vi "Trajectory Builder.vi"() -> ()   [LabVIEW 2019]
uses:
  Command Stuff/Command Editor Info.ctl
  Command Stuff/Single Cmd Info.ctl
  <vilib>/picture/picture.llb/imagedata.ctl
  <vilib>/Utility/miscctls.llb/LVPositionTypeDef.ctl
  Command Stuff/Availible Command systems for auto.ctl
  <vilib>/event_ctls.llb/lveventtype.ctl
panel:
  in  "Cluster":T1={"Path Backwards"=TRUE, "Robot Backwards"=TRUE}
  in  "Zero Vel":bool
  out "Picture":picture
  out "Duration (s)":dbl format="%#.4g"
  out "Distance (ft)":dbl format="%#.1g"
  in  "Instructions":string="Directions:\nUse mouse to ...\n    move robot position (rectangle with arrow)\n    rotate robot (red arrow)\n    move waypoints (numbered circles)\nClick in open space to add a waypoint\nShift click to delete a waypoint\nHover over a waypoint and use arrow keys to nudge\n\nTime slider and Play button will run robot along path to test for collisions.\n\nDirection and Destionation are folder selectors for files\n\nNew creates a new path at default location\n\nAppend creates a path using current path's position and heading.\n\nTo add a command, move robot using Time slider and double click Command in Palette.\n\nYou can modify command timing in the graph or Command Sequencer tree.\n\nEnable/disable a command by clicking on the enable column item.\n\nDelete a command by shift-clicking in the enable column.\n\nTo configure command parameters, Select the command name in the tree, Open Panel, enter parameters, and Inhale the parameters."
  out "WayPoints":cluster{"x":dbl, "y":dbl, "th":dbl}[](array[cluster]) {"th" format="%#_4g"}
  in  "Scale Factor":dbl=0.75
  out "Command Palette":picture
  in  "Cache":T5
  out "folder names":cluster{"name":string, "name":string}
  in  "Directory":bool
  in  "Tab Control":T6(tab)
  in  "Center Flip":bool
  in  "Snap to foot":bool
  in  "Angle Limiter":enum16{"90", "45", "15", "1"}(ring)=enum."15"
  in  "Snap robot to baseline":bool
  in  "Acceleration Overrides":T7 {"Angular \nAccelerations" step=5.0}
  in  "Sample Period (s)":dbl=0.02 format="%#_6p"
  in  "Limits":T8={"Velocity (fps)"=6.0, "Accel (fps^2)"=15.0, "Jerk (fps^3)"=150.0} {"Jerk (fps^3)" min=0.0 step=1.0; "Accel (fps^2)" min=0.0; "Velocity (fps)" min=0.0}
  in  "Conditions":T9 {"vFinal (fps)" min=0.0; "vInitial (fps)" min=0.0}
  in  "Unjank":bool
  in  "Turn Acceleration":bool=TRUE
  in  "Turn Deceleration":bool=TRUE
  in  "Open Command":bool
  in  "Inhale":bool
  in  "Command Sequence":string(tree)
  in  "Projects":u16(ring)
  in  "Refresh":bool
  in  "Time (s)":dbl(slide) scale=0.0..3.16 scale format="%#.1g"
  in  "Play":bool
  in  "Sub Dir 2":u16(ring)
  in  "Sub Dir 1":u16(ring) items=["Experimental", "Real Paths"]
  out "fps":dbl[](graph)
  in  "Append":bool
  in  "Open":i32(listbox)
  in  "Filename":string
  in  "Save":bool
  in  "New":bool
  # "Command Palette"
  # "Power Port"
  # "Feeder Station"
  # "Nicotine"
  # "Interaction Options"
  # "1"
  # "2"
  # "3"
  # "4"
  # "5"
  # "6"
  # "7"
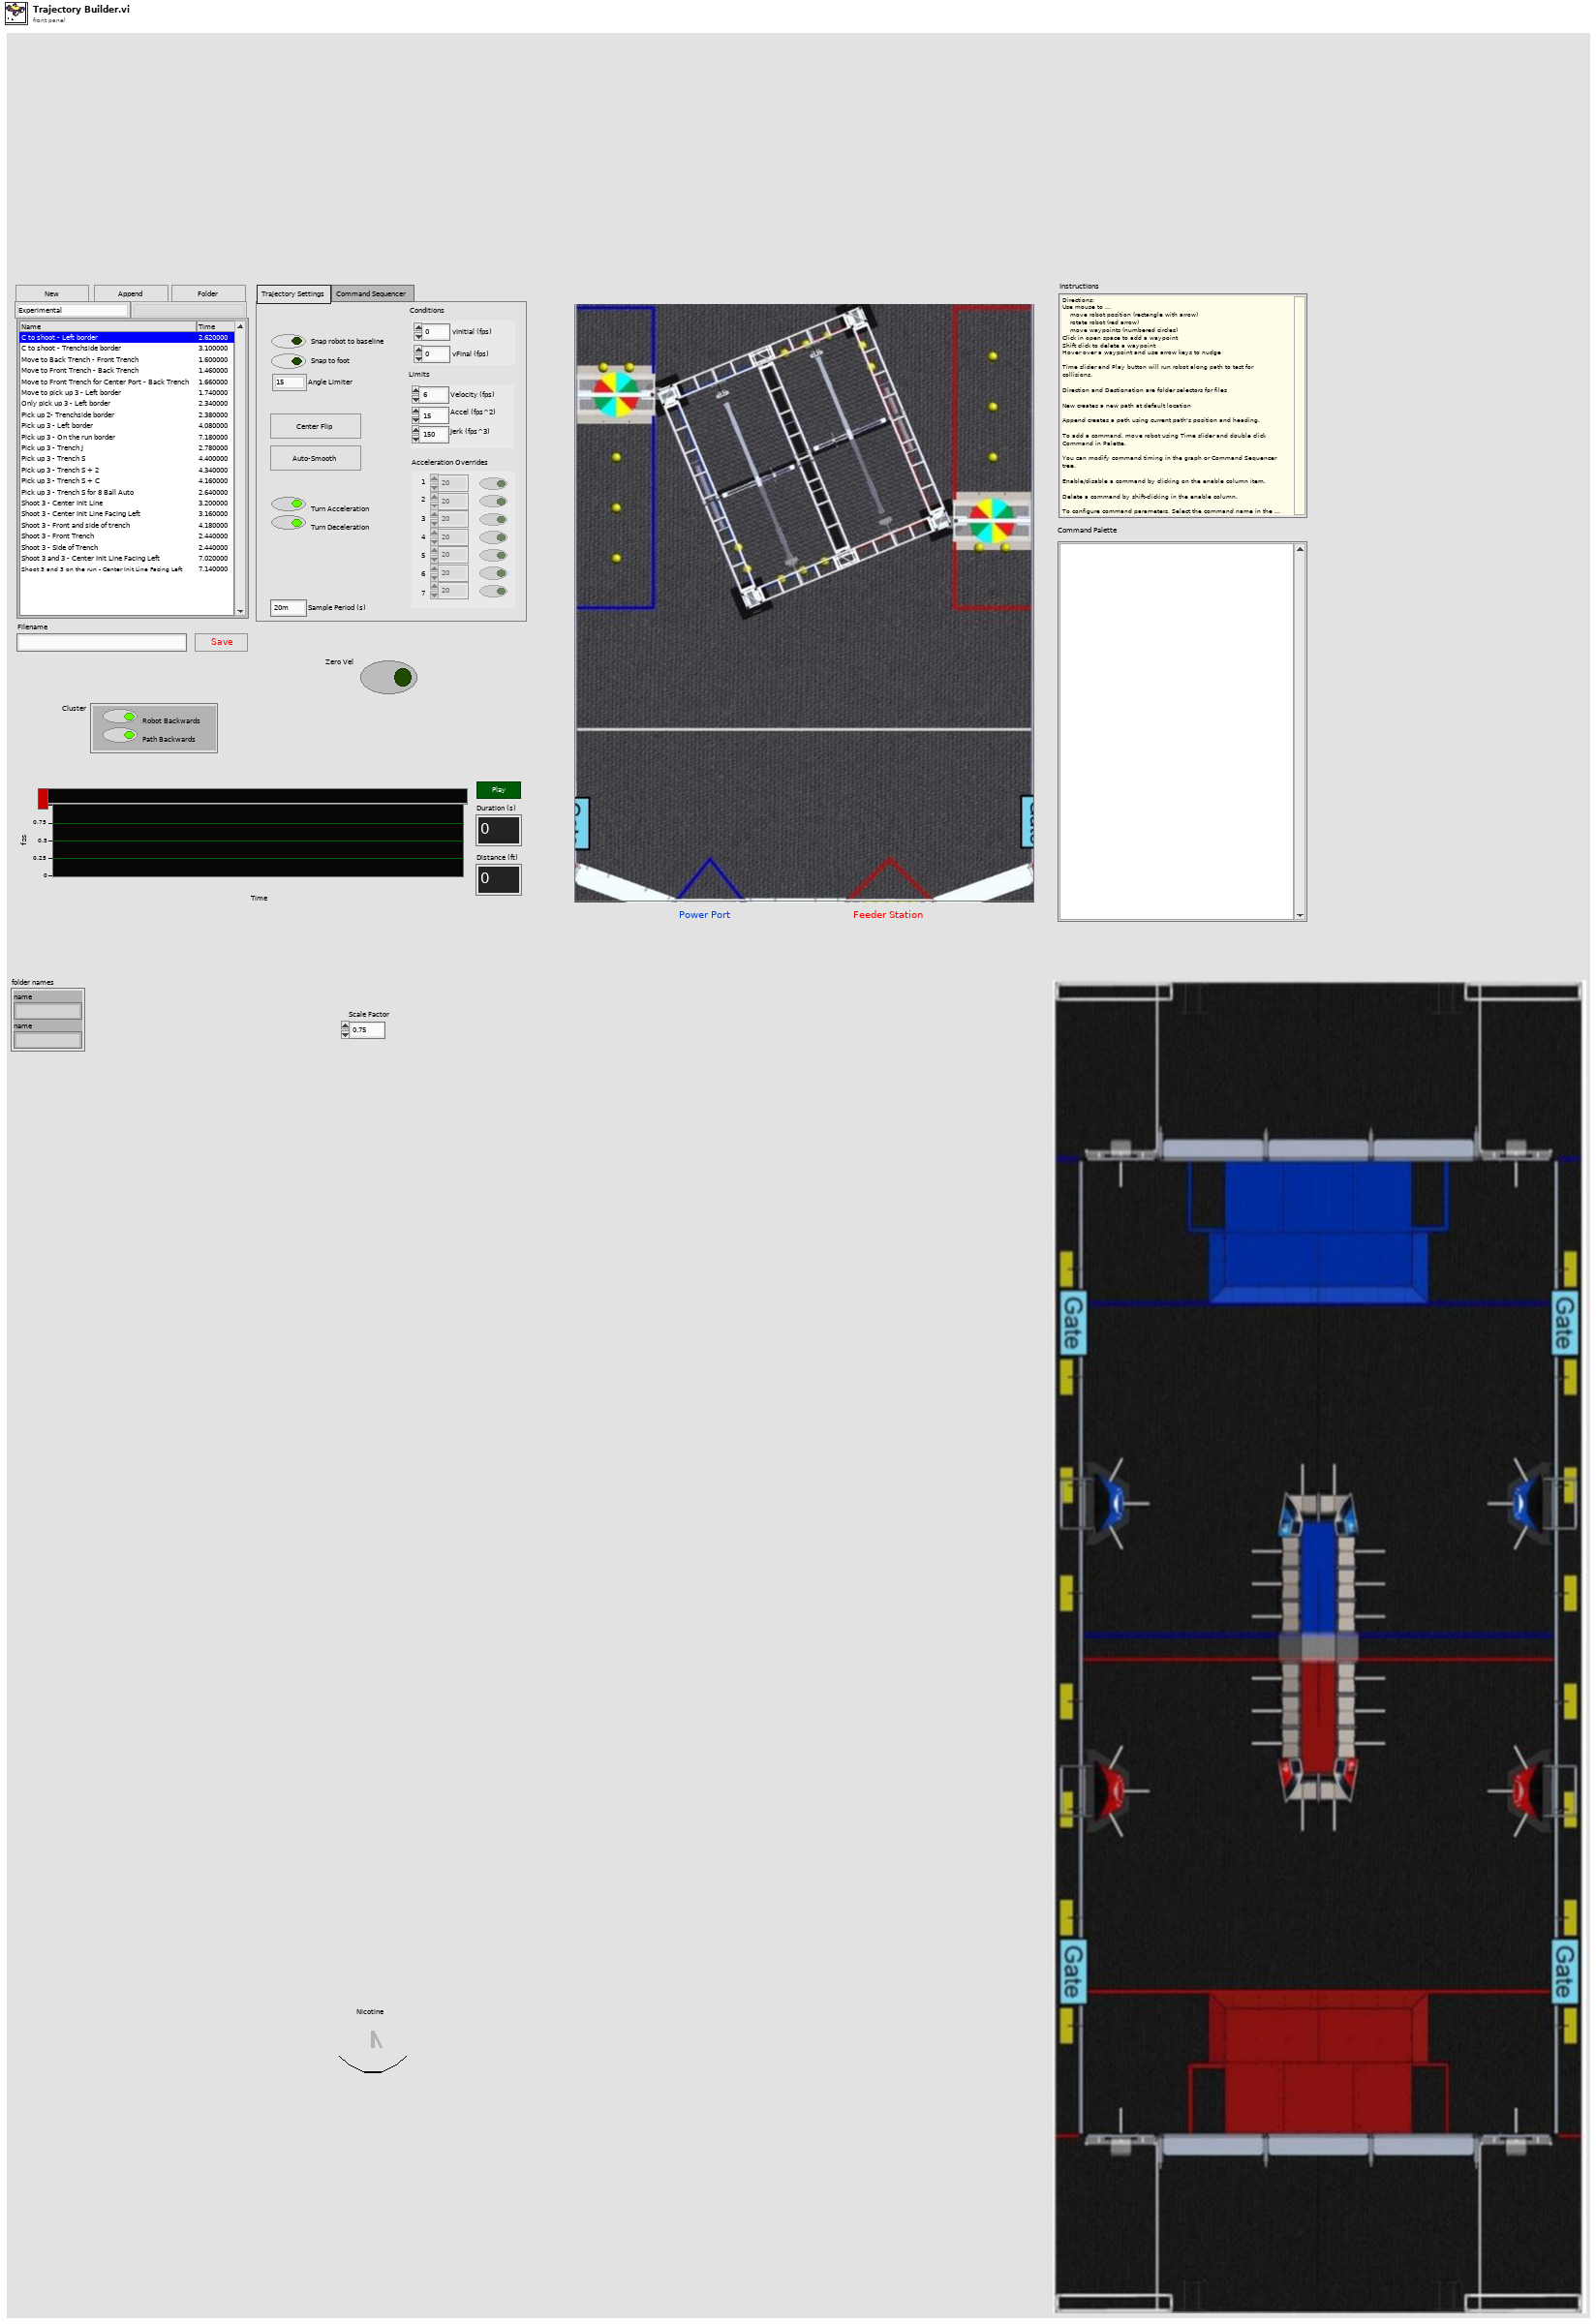
[diagram p1: front panel]
types:
  T1 = cluster{"Path Backwards":bool, "Robot Backwards":bool}
  T2 = typedef "Command Editor Info.ctl" = T3[]
  T3 = typedef "Single Cmd Info.ctl" = cluster{"Name":string, "CPTM.DataType":variant, "All Control Values Variant":cluster{"Name":string, "Variant Data":variant}[], "icon full":T4, "icon scaled":T4, "Path":path, "Subsystem Color":u32}
  T4 = typedef "imagedata.ctl" = cluster{"image type":i32, "image depth":i32, "image":u8[], "mask":u8[], "colors":u32[], "Rectangle":cluster{"left":i16, "top":i16, "right":i16, "bottom":i16}}
  T5 = cluster{"Filtered Command Info Out":T2, "2D Picture":picture}
  T6 = enum32{"Trajectory Settings", "Command Sequencer"}
  T7 = cluster{"Angular \nAccelerations":dbl[], "Accel Override Bools":bool[]}
  T8 = cluster{"Velocity (fps)":dbl, "Accel (fps^2)":dbl, "Jerk (fps^3)":dbl}
  T9 = cluster{"vInitial (fps)":dbl, "vFinal (fps)":dbl}
  T10 = typedef "LVPositionTypeDef.ctl" = cluster{"Left":i32, "Top":i32}
  T11 = cluster{"Sample Period (s)":dbl, "Limits":cluster{"Velocity (fps)":dbl, "Acceleration (fps^2)":dbl, "Jerk (fps^3)":dbl}, "Conditions":cluster{"vInitial (fps)":dbl, "vFinal (fps)":dbl}, "output cluster":cluster{"Angular \nAccelerations":dbl[], "Override Limits?":bool[]}}
  T12 = cluster{"Segment Name":string, "Type":enum16{"Accel Straight", "Const Straight", "Blend", "Circle"}, "Traj Pos Points":cluster{"x":dbl, "y":dbl, "th":dbl}[], "Traj Vel Points":cluster{"V":dbl, "th":dbl}[], "Accel Index":i32, "Decel Index":i32}[]
  T13 = cluster{"Angular \nAccelerations":dbl[], "Override Limits?":bool[]}
  T14 = cluster{"Index":i32, "Pt Test Results":enum16{"Miss", "Rect Hit", "Arrow Hit"}}
  T15 = cluster{"Drag Object":cluster{"Index":i32, "x":dbl, "y":dbl}, "Hover Object":cluster{"Index":i32, "Pt Test Results":enum16{"Miss", "Rect Hit", "Arrow Hit"}}, "Filename":string}
  T16 = cluster{"Trajectory Data":cluster{"Segment Name":string, "Type":enum16{"Accel Straight", "Const Straight", "Blend", "Circle"}, "Traj Pos Points":cluster{"x":dbl, "y":dbl, "th":dbl}[], "Traj Vel Points":cluster{"V":dbl, "th":dbl}[], "Accel Index":i32, "Decel Index":i32}[], "Points":cluster{"x":dbl, "y":dbl, "th":dbl}[], "Cluster":cluster{"Sample Period (s)":dbl, "Limits":cluster{"Velocity (fps)":dbl, "Acceleration (fps^2)":dbl, "Jerk (fps^3)":dbl}, "Conditions":cluster{"vInitial (fps)":dbl, "vFinal (fps)":dbl}, "output cluster":cluster{"Angular \nAccelerations":dbl[], "Override Limits?":bool[]}}, cluster{"Time (s)":dbl, T3, bool}[]}
  T17 = cluster{"Velocity":dbl, "Sample Time":dbl, "Accel":dbl}
  T18 = cluster{"Sample Period (s)":dbl, "Limits":cluster{"Velocity (fps)":dbl, "Acceleration (fps^2)":dbl, "Jerk (fps^3)":dbl}, "Conditions":cluster{"vInitial (fps)":dbl, "vFinal (fps)":dbl}}
  T19 = cluster{"Sample Period (s)":dbl, "Limits":cluster{"Velocity (fps)":dbl, "Acceleration (fps^2)":dbl, "Jerk (fps^3)":dbl}, "Conditions":cluster{"vInitial (fps)":dbl, "vFinal (fps)":dbl}, "Min Rads":dbl[]}
  T20 = typedef "Availible Command systems for auto.ctl" = u16
  T21 = cluster{"Time into Path":dbl, "System":T20, "Item Selected?":bool, "System Selection":T20}[]
  T22 = typedef "lveventtype.ctl" = enum32{"Null", "Timeout", "Annotation Menu Selection", "Annotation Menu Selection?", "App Instance Close", "App Instance Close?", "Autoscale Range Change", "Bookmark Info Change", "Cell Edit", "Cell Edit?", "Cursor Grab", "Cursor Grab?", "Cursor Menu Selection", "Cursor Menu Selection?", "Cursor Move", "Cursor Release", "Data Change", "Direction Change", "Display State Change", "Drag Ended", "Drag Enter", "Drag Leave", "Drag Over", "Drag Source Update", "Drag Starting", "Drag Starting?", "Drop", "Exec State Change", "Key Down", "Key Down?", "Key Repeat", "Key Repeat?", "Key Up", "Listbox Double Click", "Menu Activation?", "Menu Selection (App)", "Menu Selection? (App)", "Menu Selection (User)", "Mouse Down", "Mouse Down?", "Mouse Enter", "Mouse Leave", "Mouse Move", "Mouse Up", "Mouse Wheel", "NI Security User Change (App)", "Pane Size", "Panel Close", "Panel Close?", "Panel Resize", "Plot Attribute Change", "Scale Range Change", "Shortcut Menu Activation?", "Shortcut Menu Selection (App)", "Shortcut Menu Selection? (App)", "Shortcut Menu Selection (User)", "Tree Double Click", "Tree Drag", "Tree Drag?", "Tree Drop", "Tree Drop?", "Tree Item Close", "Tree Item Close?", "Tree Item Open", "Tree Item Open?", "User Event", "Value Change"}
  T23 = enum32{"Invalid", "Standard", "Closed", "Hidden", "Minimized", "Maximized"}
  T24 = cluster{"Sample Period (s)":dbl, "Limits":cluster{"Velocity (fps)":dbl, "Accel (fps^2)":dbl, "Jerk (fps^3)":dbl}, "Conditions":cluster{"vInitial (fps)":dbl, "vFinal (fps)":dbl}, " Acceleration Overrides":cluster{"Angular \nAccelerations":dbl[], "Accel Override Bools":bool[]}}
  T25 = cluster{"Segment Name":string, "Type":enum16{"Accel Straight", "Const Straight", "Blend", "Circle"}, "Traj Pos Points":cluster{"x":dbl, "y":dbl, "th":dbl}[], "Traj Vel Points":cluster{"V":dbl, "th":dbl}[], "Accel Index":i32, "Decel Index":i32}
  T26 = cluster{"Trajectory Data":cluster{"Segment Name":string, "Type":enum16{"Accel Straight", "Const Straight", "Blend", "Circle"}, "Traj Pos Points":cluster{"x":dbl, "y":dbl, "th":dbl}[], "Traj Vel Points":cluster{"V":dbl, "th":dbl}[], "Accel Index":i32, "Decel Index":i32}[], "Updated Waypoints":cluster{"x":dbl, "y":dbl, "th":dbl}[], "Cluster":cluster{"Sample Period (s)":dbl, "Limits":cluster{"Velocity (fps)":dbl, "Accel (fps^2)":dbl, "Jerk (fps^3)":dbl}, "Conditions":cluster{"vInitial (fps)":dbl, "vFinal (fps)":dbl}, " Acceleration Overrides":cluster{"Angular \nAccelerations":dbl[], "Accel Override Bools":bool[]}}, cluster{"Time (s)":dbl, T3, bool}[]}
  T27 = cluster{"Velocity":dbl, "Accel":dbl, "Accel":dbl}
  T28 = cluster{"Velocity (fps)":dbl, "Acceleration (fps^2)":dbl, "Jerk (fps^3)":dbl}
  T29 = cluster{"Trajectory Data":cluster{"Segment Name":string, "Type":enum16{"Accel Straight", "Const Straight", "Blend", "Circle"}, "Traj Pos Points":cluster{"x":dbl, "y":dbl, "th":dbl}[], "Traj Vel Points":cluster{"V":dbl, "th":dbl}[], "Accel Index":i32, "Decel Index":i32}[], "Points":cluster{"x":dbl, "y":dbl, "th":dbl}[], cluster{"Sample Period (s)":dbl, "Limits":cluster{"Velocity (fps)":dbl, "Accel (fps^2)":dbl, "Jerk (fps^3)":dbl}, "Conditions":cluster{"vInitial (fps)":dbl, "vFinal (fps)":dbl}, " Acceleration Overrides":cluster{"Angular \nAccelerations":dbl[], "Accel Override Bools":bool[]}}, cluster{"Time (s)":dbl, T3, bool}[]}
  T30 = typedef "LVPoint32TypeDef.ctl" = cluster{"Horizontal":i32, "Vertical":i32}
  T31 = cluster{"Shift":bool, "Ctrl":bool, "Alt":bool, "Cmd":bool, "Opt":bool}
  T32 = typedef "LVBoundsTypeDef.ctl" = cluster{"Width":u32, "Height":u32}
  T33 = cluster{"Snap robot to baseline":bool, "Snap to foot":bool, "Angle Limiter":enum16{"90", "45", "15", "1"}}
  T34 = cluster{i32, "Pt Test Results":enum16{"Miss", "Rect Hit", "Arrow Hit"}}
  T35 = typedef "eventvkey.ctl" = enum16{"ASCII", "Enter", "Return", "Shift", "Ctrl", "Alt", "Cmd", "Opt", "Caps", "NumLock", "Clear", "Break", "Up", "Down", "Left", "Right", "Insert", "Delete", "Home", "End", "PageUp", "PageDown", "Escape", "Help", "Pause", "ScrollLock", "F1", "F2", "F3", "F4", "F5", "F6", "F7", "F8", "F9", "F10", "F11", "F12", "F13", "F14", "F15", "F16", "F17", "F18", "F19", "F20", "F21", "F22", "F23", "F24", "Play", "VolumeUp", "VolumeDown", "Mute", "Two Byte Char"}
  T36 = cluster{"Name":string, "CPTM.DataType":variant, "Get All Control Values Variant":cluster{"Name":string, "Variant Data":variant}[], "Color 256":T4, "Subsystem Color":u32}[]
  T37 = cluster{"Trajectory Data":cluster{"Segment Name":string, "Type":enum16{"Accel Straight", "Const Straight", "Blend", "Circle"}, "Traj Pos Points":cluster{"x":dbl, "y":dbl, "th":dbl}[], "Traj Vel Points":cluster{"V":dbl, "th":dbl}[], "Accel Index":i32, "Decel Index":i32}[], "Updated Waypoints":cluster{"x":dbl, "y":dbl, "th":dbl}[], cluster{"Sample Period (s)":dbl, "Limits":cluster{"Velocity (fps)":dbl, "Accel (fps^2)":dbl, "Jerk (fps^3)":dbl}, "Conditions":cluster{"vInitial (fps)":dbl, "vFinal (fps)":dbl}, " Acceleration Overrides":cluster{"Angular \nAccelerations":dbl[], "Accel Override Bools":bool[]}}, cluster{"Time (s)":dbl, T3, bool}[]}
  T38 = cluster{"Horizontal":dbl, "Vertical":dbl, "th":dbl}
  T39 = cluster{"Name":string, "Color":u32, "Style":i32, "Point Style":i32, "Name Visible":bool, "Allow Drag":bool, "Annotation Mode":i32, "Plot":i32, "Index":i32, "Position":cluster{"X":dbl, "Y":dbl}, "X Scale":i32, "Y Scale":u32, "Show Arrow":bool, "Lock Name":bool, "Plot Area":i32, "Label Offset":cluster{"X":dbl, "Y":dbl}}[]
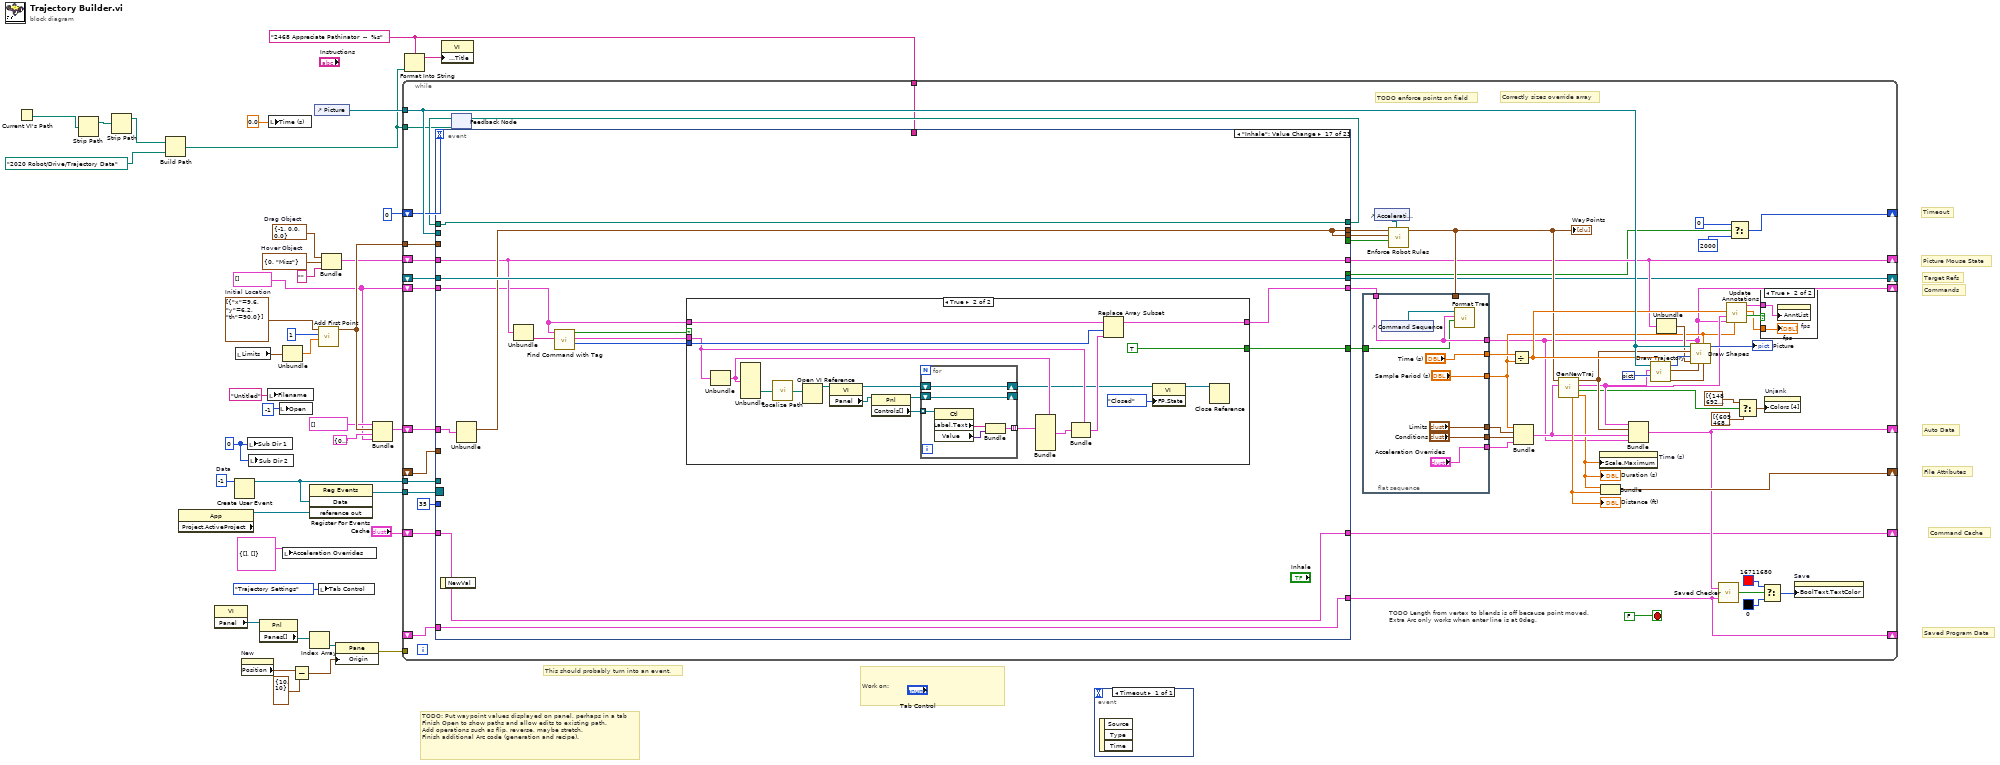
[diagram p0: block diagram]
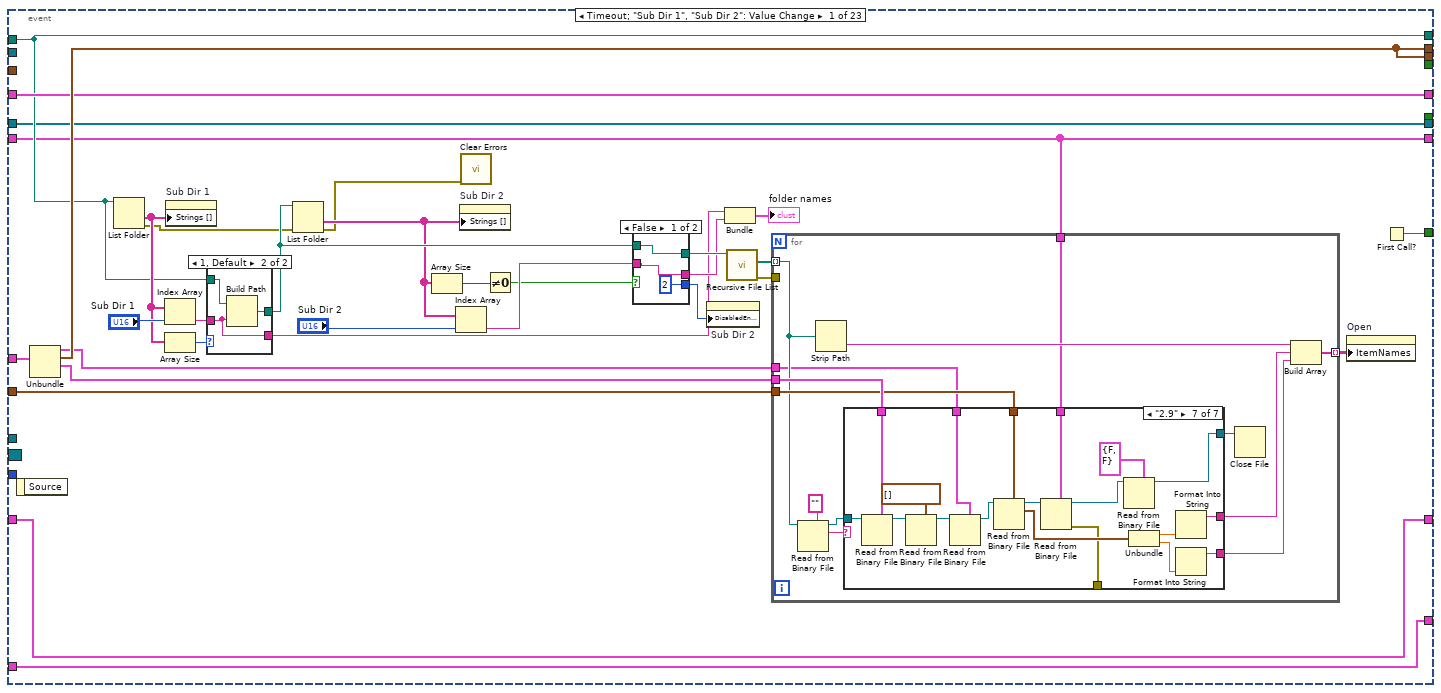
[diagram p3: hidden frame]
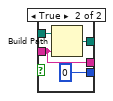
[diagram p5: hidden frame]
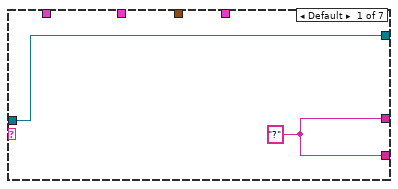
[diagram p6: hidden frame]
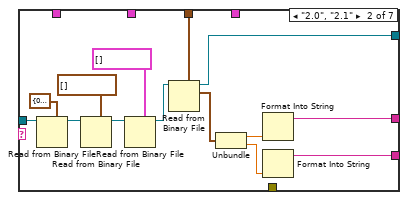
[diagram p7: hidden frame]
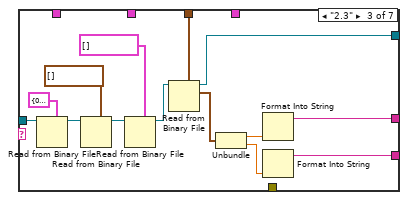
[diagram p8: hidden frame]
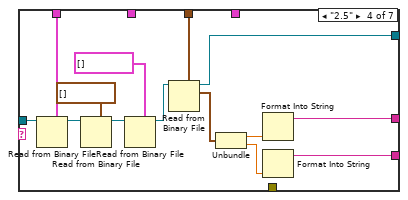
[diagram p9: hidden frame]
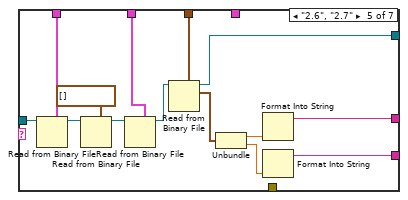
[diagram p10: hidden frame]
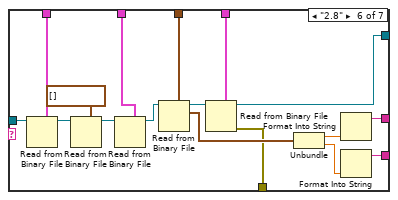
[diagram p11: hidden frame]
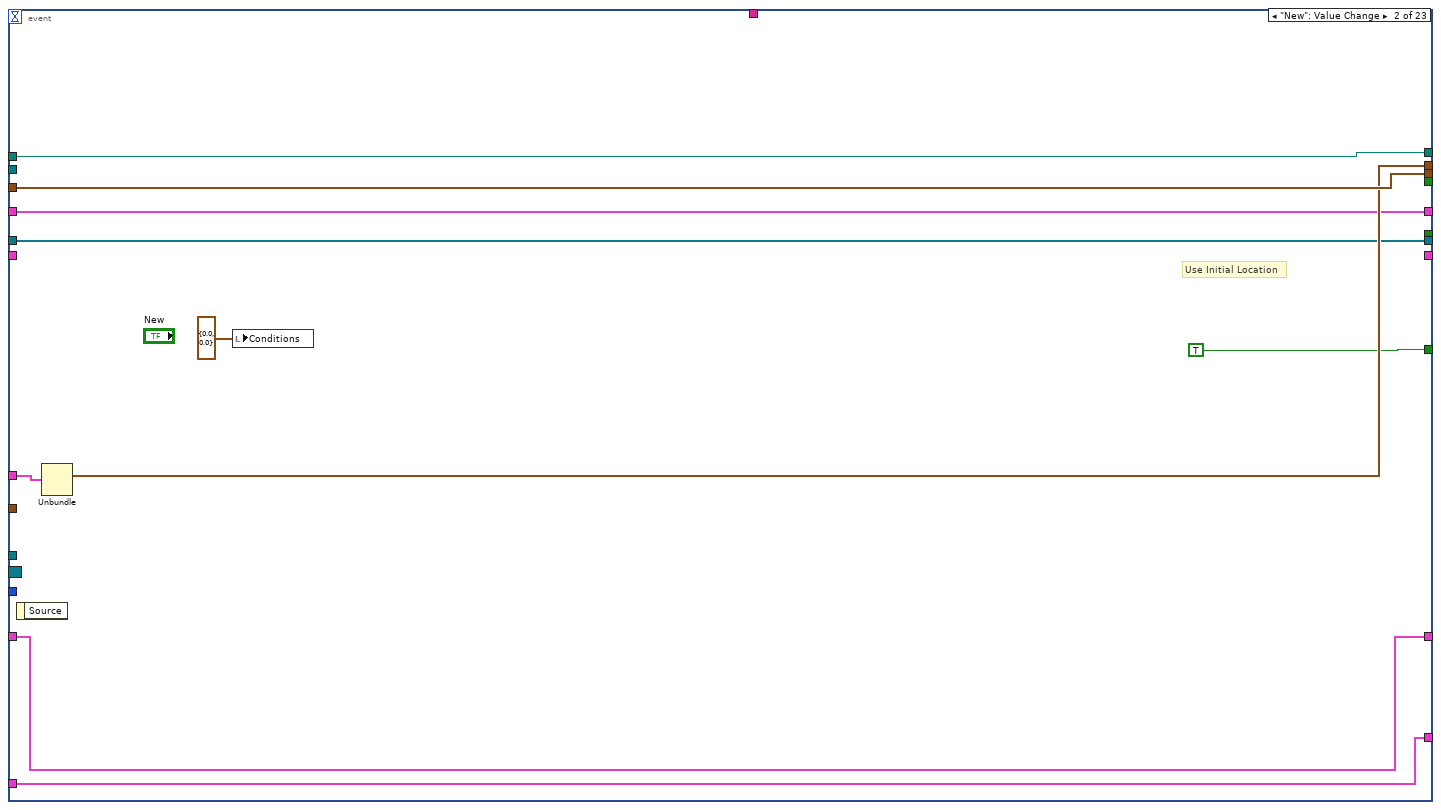
[diagram p12: hidden frame]
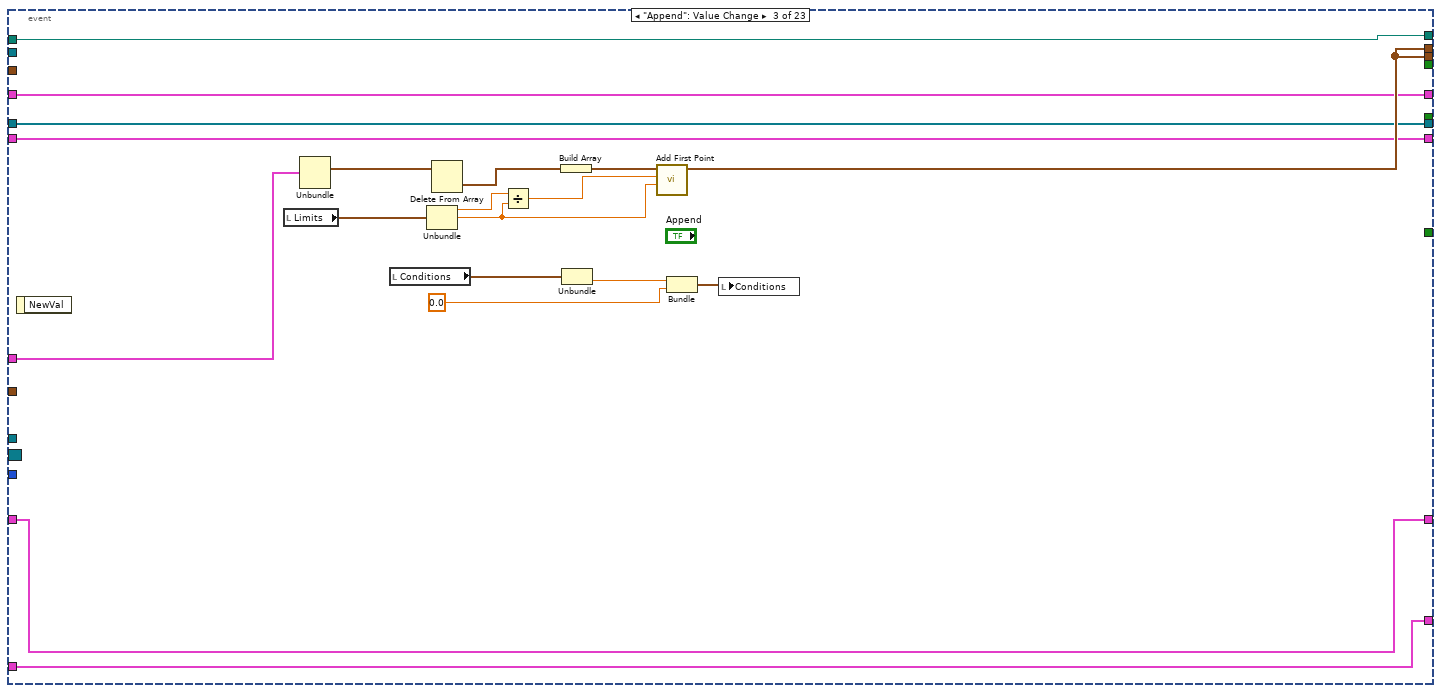
[diagram p13: hidden frame]
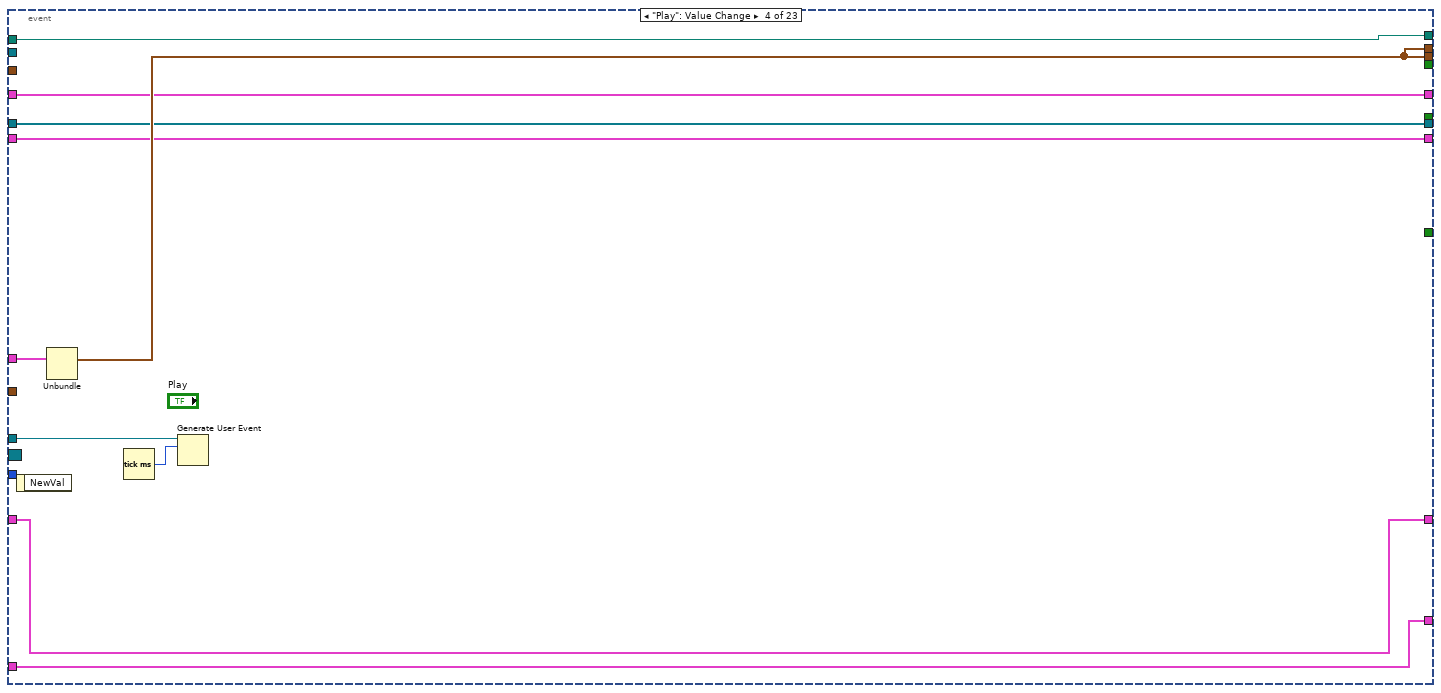
[diagram p14: hidden frame]
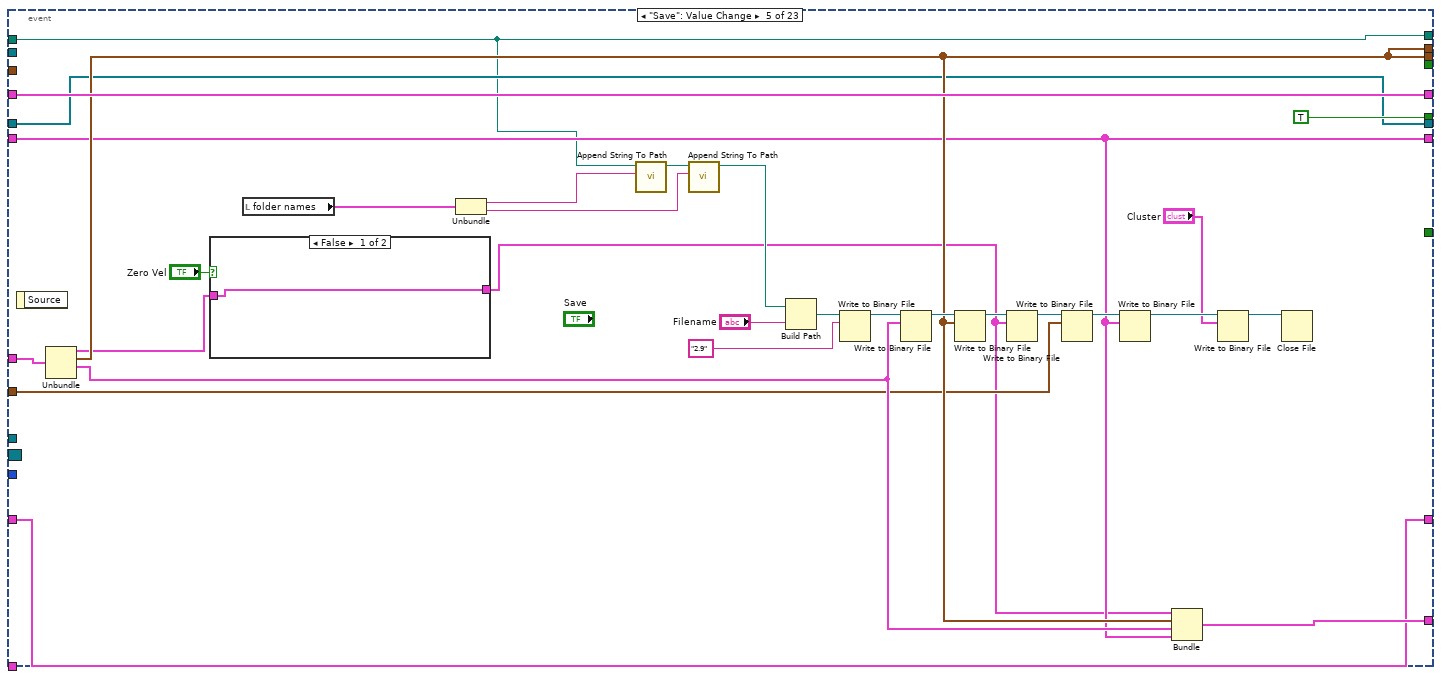
[diagram p15: hidden frame]
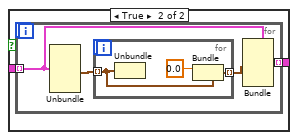
[diagram p16: hidden frame]
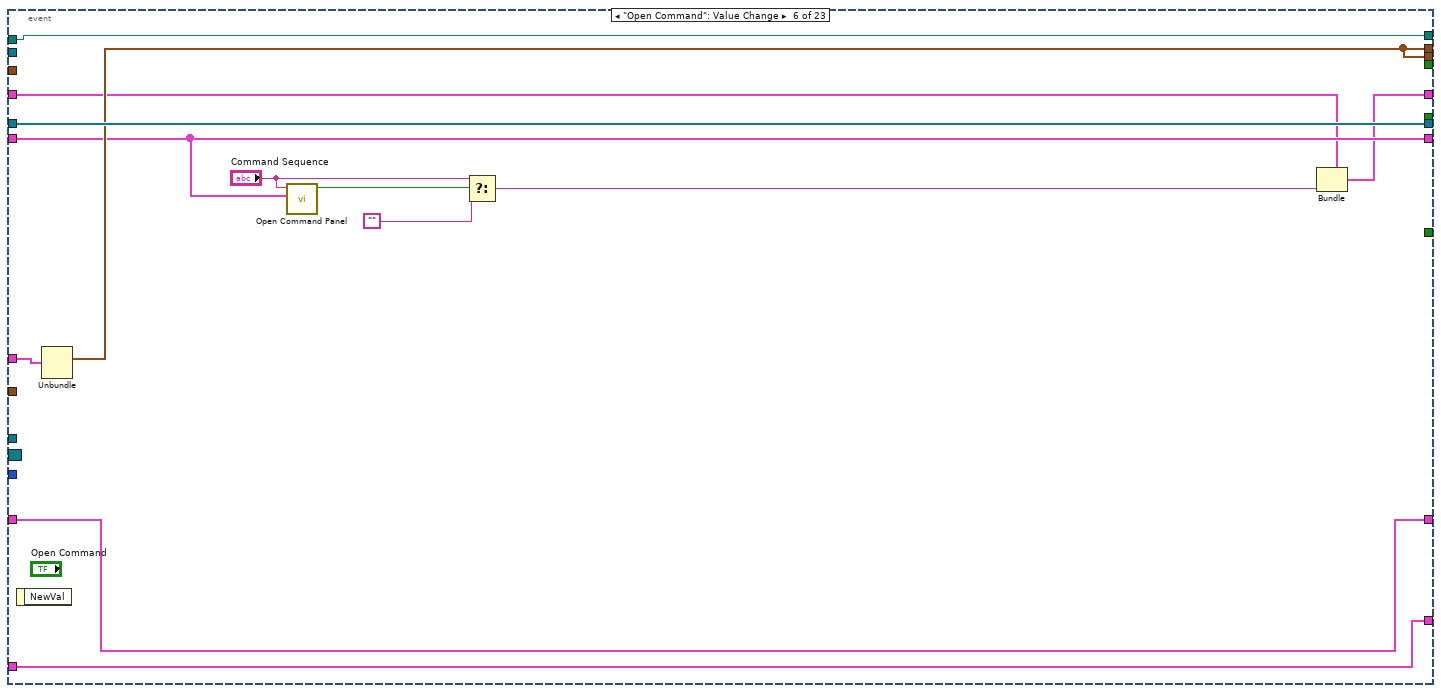
[diagram p17: hidden frame]
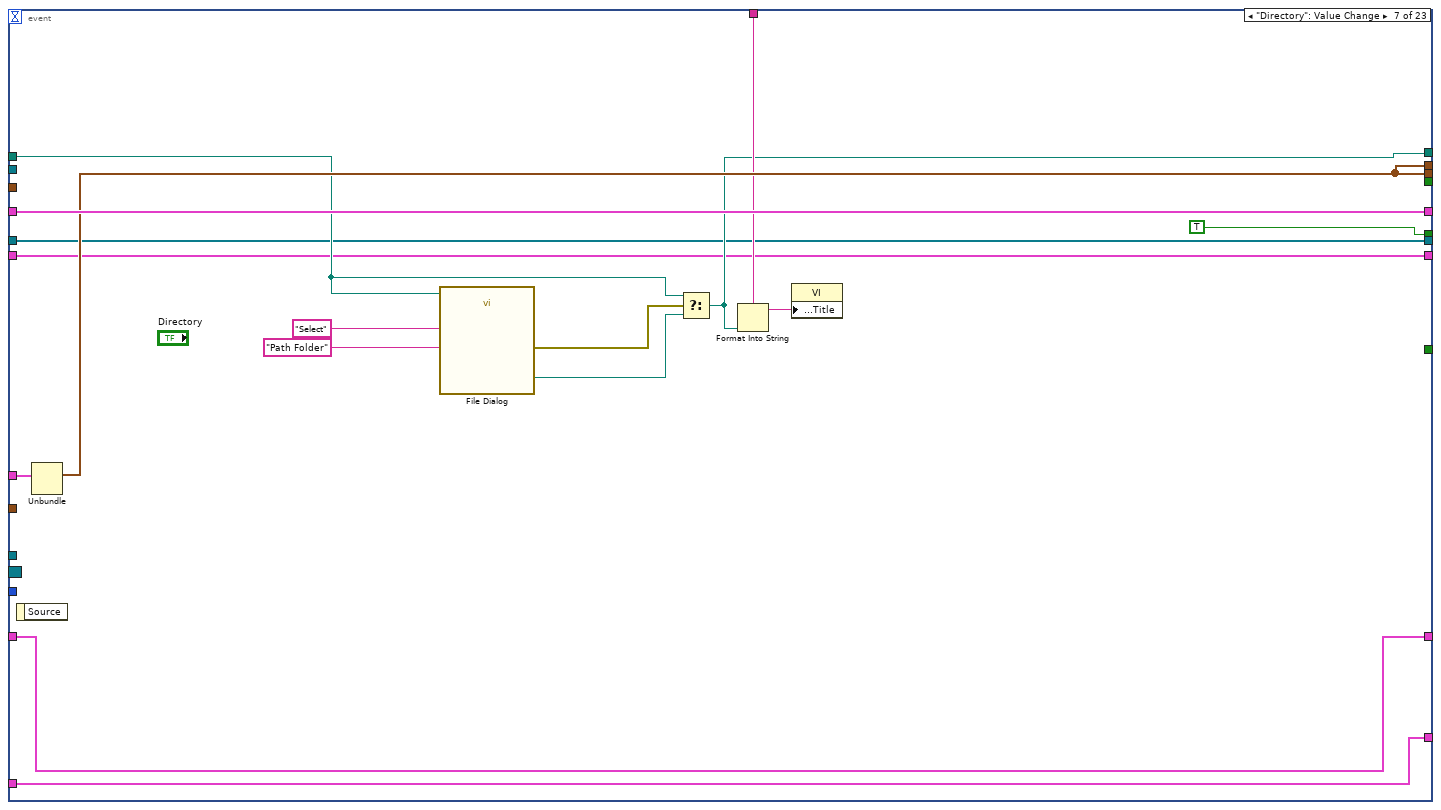
[diagram p18: hidden frame]
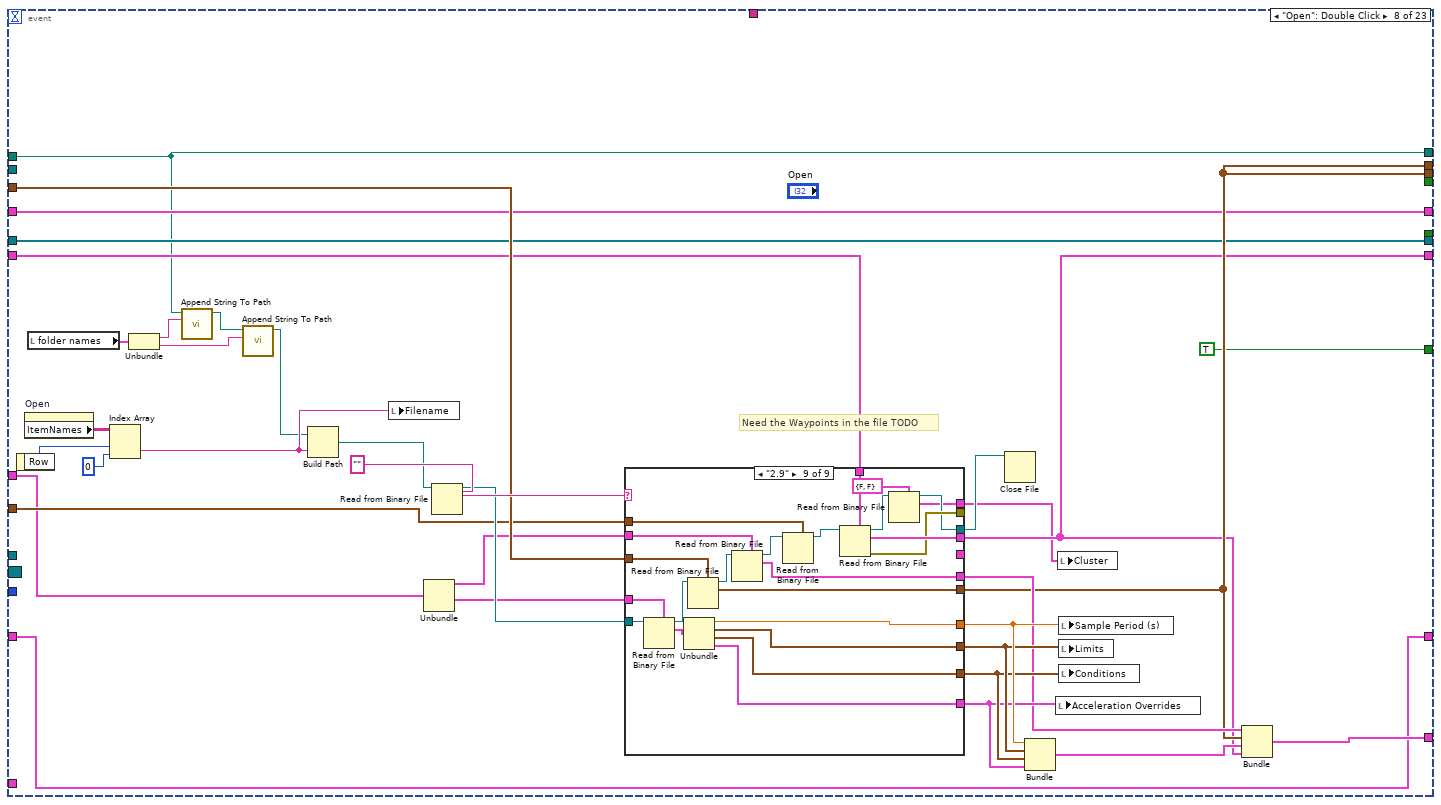
[diagram p19: hidden frame]
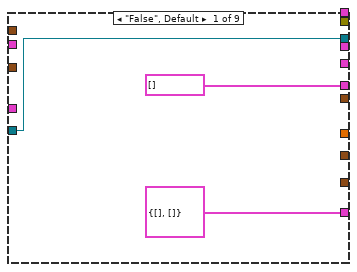
[diagram p20: hidden frame]
diagram:
  w6 = cluster{"Time (s)":dbl, T3, bool}[] []
  w18 = 0 ("th")
  w19 = "2468 Appreciate Pathinator  --  %s" ("format string")
  w29 = -1  # Data
  w23 = T14 {"Index"=0, "Pt Test Results"=enum."Miss"}  # Hover Object
  w22 = cluster{"Index":i32, "x":dbl, "y":dbl} {"Index"=-1, "x"=0.0, "y"=0.0}  # Drag Object
  w38 = cluster{"x":dbl, "y":dbl, "th":dbl}[] [{"x"=9.6, "y"=6.2, "th"=90.0}]  # Initial Location
  # "Saved Program Data"
  # "Command Cache"
  # "File Attributes"
  # "Commands"
  # "Target Refs"
  # "Picture Mouse State"
  # "Auto Data"
  # "Timeout"
  # "This should probably turn into an event."
  # "Work on:"
  # "TODO: Put waypoint values displayed on panel, perhaps in a tab\nFinish Open to show paths and allow edits to existing path.\nAdd operations such as flip, reverse, maybe stretch.\nFinish additional Arc code (generation and recipe)."
  n1 = Current VI's Path() -> (path=w5:path)
  n2 = Strip Path(path=w5) -> (stripped path=w4:path)  [unwired: 1 out]
  n3 = Strip Path(path=w4) -> (stripped path=w3:path)  [unwired: 1 out]
  n4 = Build Path(base path=w3, name or relative path=path "2020 Robot/Drive/Trajectory Data" ("Robot File")) -> (appended path=w1:path)
  n5 = property class="App" props=["Project.ActiveProject"]() -> (reference out=w7:refnum<vi>)  [unwired: 2 in, 2 out]
  n6 = property class="VI"() -> ("Panel"=w15:refnum<vi>)  [unwired: 2 in, 2 out]
  n7 = Create User Event(user event datatype=w29) -> (user event=w30:refnum<user-event>)  [unwired: 1 in, 1 out]
  n8 = local read "Limits"() -> (w35:T8)
  n9 = property on="New" class="Bool"() -> ("Position"=w11:T10)  [unwired: 2 in, 2 out]
  n10 = local write "Sub Dir 1"(w18) -> ()
  n11 = local write "Sub Dir 2"(w18) -> ()
  n12 = property class="Pnl"(reference=w15) -> ("Panes[]"=w14:refnum<vi>[])  [unwired: 1 in, 2 out]
  n13 = local write "Filename"("Untitled" ("Filename")) -> ()
  n14 = local write "Time (s)"(0.0 ("Time")) -> ()
  n15 = local write "Open"(-1) -> ()
  n16 = Unbundle(w35) -> ("Accel (fps^2)"=w34:dbl)  [unwired: 2 out]
  n17 = local write "Acceleration Overrides"(T13 {"Angular \nAccelerations"=[], "Override Limits?"=[]} ("Angular Accelerations")) -> ()
  n18 = Subtract(x=w11, y=T10 {"Left"=10, "Top"=10}) -> (x-y=w10:T10)
  n19 = register-events(w30, w7) -> (reference out=w31:refnum<event-registration>)  [unwired: 2 in, 1 out]
  n20 = Index Array(array=w14) -> (element=w13:refnum<vi>)  [unwired: 1 in]
  n21 = control-ref of="Picture"() -> (w40:refnum<vi>)
  n22 = call "Add First Point.vi"("Accel (f/s^2)"=w34, "Time (s)"=1 ("th"), "Initial Points"=w38) -> ("Points"=w27:cluster{"x":dbl, "y":dbl, "th":dbl}[])  [unwired: 8 in]
  n23 = local write "Tab Control"(T6."Trajectory Settings" ("Tab Control")) -> ()
  n24 = Bundle("Drag Object"=w22, "Hover Object"=w23, "Filename"="") -> (w21:T15)  [unwired: 1 in]
  n25 = property class="Pane"(reference=w13, "Origin"=w10) -> (error out=w9:errorcluster)  [unwired: 1 in, 1 out]
  n26 = Bundle("Trajectory Data"=T12 [], "Points"=w27, "Cluster"=T11 {"Sample Period (s)"=0.02, "Limits"={"Velocity (fps)"=11.0, "Acceleration (fps^2)"=19.0, "Jerk (fps^3)"=150.0}, "Conditions"={"vInitial (fps)"=0.0, "vFinal (fps)"=0.0}, "output cluster"={"Angular \nAccelerations"=[], "Override Limits?"=[]}}, w6) -> (w26:T16)  [unwired: 1 in]
  n27 = while {
    tunnel: w27 -> [w103]
    tunnel: w40 -> [w102]
    shift-right: [w62] -> _
    shift-left: 0 -> [w96]
    shift-right: [w95] -> _
    shift-left: _ -> [w94]
    tunnel: w1 -> [w75]
    tunnel: w31 -> [w88]
    tunnel: w30 -> [w87]
    shift-right: [w85] -> _
    shift-left: _ -> [w86]
    shift-right: [w74] -> _
    shift-left: w26 -> [w73]
    shift-right: [w67] -> _
    shift-left: w21 -> [w68]
    tunnel: w19 -> [w65]
    shift-right: [w55] -> _
    shift-left: _ -> [w54]
    shift-right: [w52] -> _
    shift-left: "Cache" -> [w53]
    shift-right: [w45] -> _
    shift-left: w6 -> [w50]
    tunnel: w9 -> [_]
    stop <- FALSE stop-if-true
    # "Correctly sizes override array"
    # "TODO Length from vertex to blends is off because point moved.\nExtra Arc only works when enter line is at 0deg."
    # "TODO enforce points on field"
    n28 = feedback #1(w75) -> (w76:path)
    n29 = event shown="[16] \"Inhale\": Value Change" {
      selector: w88 -> [_ _ _ _ _ _ _ _ _ _ _ _ _ _ _ _ _ _ _ _ _ _ _]
      dyn-events: _ -> [_ _ _ _ _ _ _ _ _ _ _ _ _ _ _ _ _ _ _ _ _ _ _]
      timeout: w96 -> [_ _ _ _ _ _ _ _ _ _ _ _ _ _ _ _ _ _ _ _ _ _ _]
      tunnel: [w128 w275 w293 w299 w322 w353 w370 w390 w574 w677 w721 w758 w782 w808 w827 w847 w883 w921 w955 w1003 w1028 w1060 w1091] -> w93
      tunnel: w103 -> [_ w275 _ _ _ _ _ w402 _ _ _ _ _ _ _ _ _ _ _ _ _ _ _]
      tunnel: w102 -> [_ _ _ _ _ _ _ _ w573 w660 _ w745 _ _ _ _ _ _ _ _ _ _ _]
      tunnel: w76 -> [w126 w273 w282 w304 w315 w357 w364 w377 w571 w671 w716 w759 w798 w811 w829 w851 w887 w927 w960 w1007 w1033 w1065 w1096]
      tunnel: [w128 w270 w293 w299 w322 w353 w370 w390 w568 w668 w712 w743 w782 w808 w827 w847 w883 w921 w955 w1003 w1028 w1060 w1091] -> w92
      tunnel: w94 -> [w144 _ _ _ w318 _ _ w400 _ _ _ _ _ _ _ _ _ _ _ _ _ _ _]
      tunnel: [_ _ _ _ _ _ _ _ _ _ TRUE ("Flip Over Center") _ _ _ _ _ _ _ _ _ _ _ _] -> w91
      tunnel: [w126 w273 w282 w304 w315 w357 w362 w377 w571 w671 w716 w759 w798 w811 w829 w851 w887 w927 w960 w1007 w1033 w1065 w1096] -> w77
      tunnel: w87 -> [_ _ _ w303 _ _ _ _ _ _ _ _ w797 _ _ _ _ _ _ _ _ _ _]
      tunnel: [w137 w272 w283 w302 w327 w356 w372 w392 w570 w670 w715 w746 w794 w810 w830 w850 w886 w926 w959 w1006 w1032 w1064 w1095] -> w85
      tunnel: w86 -> [w137 w272 w283 w302 _ w356 w372 _ w570 w670 w715 w746 w794 w810 w830 w850 w886 w926 w959 w1006 w1032 w1064 w1095]
      tunnel: w73 -> [w130 w271 w281 w300 w325 w354 w371 w389 w569 w669 w713 w744 w783 w809 w828 w848 w884 w923 w956 w1004 w1029 w1061 w1092]
      tunnel: w68 -> [w127 w269 w279 w298 w323 w350 w373 w387 w565 w661 w711 w741 w781 w807 w826 w846 w882 w925 w958 w989 w1031 w1063 w1094]
      tunnel: [w127 w269 w279 w298 w323 w351 w373 w387 w567 w665 w711 w741 w781 w807 w826 w846 w882 w925 w958 w990 w1031 w1063 w1094] -> w67
      tunnel: w65 -> [_ _ _ _ _ _ w367 _ _ _ _ _ _ _ _ _ _ _ _ _ _ _ _]
      tunnel: [_ _ _ _ TRUE _ TRUE _ _ _ _ _ _ _ _ _ _ _ _ _ _ _ _] -> w61
      tunnel: [w123 w267 w278 w297 w320 w355 w361 w384 w561 w663 w708 w739 w780 w805 w825 w849 w885 w924 w957 w1005 w1030 w1062 w1093] -> w55
      tunnel: w54 -> [w123 w267 w278 w297 w320 w355 w361 w384 w561 w663 w708 w739 w780 w804 w825 w849 w885 w924 w957 w1005 w1030 w1062 w1093]
      tunnel: w53 -> [w120 w268 w277 w296 w319 w345 w360 w383 w563 w662 w707 w738 w779 w803 _ w831 w874 w914 w940 w987 w1013 w1051 w1078]
      tunnel: [w120 w268 w277 w296 w319 w345 w360 w383 w563 w662 w707 w738 w779 w803 w819 w831 w874 w914 w940 w987 w1013 w1051 w1078] -> w52
      tunnel: 35 -> [_ _ _ _ _ _ _ _ _ _ _ _ _ _ _ _ _ _ _ _ _ w1053 w1087]
      tunnel: w50 -> [w118 _ w276 w295 w317 w352 w358 w381 w562 w659 w706 w737 w778 w802 w818 w832 w876 w919 w943 w992 w1016 w1052 w1080]
      tunnel: [w118 _ w276 w295 w317 w352 w358 w380 w562 w659 w706 w737 w778 w802 w818 w832 w877 w920 w941 w992 w1017 w1052 w1081] -> w49
      tunnel: [w117 TRUE _ _ _ _ _ TRUE _ _ _ _ _ _ _ w839 w875 TRUE w942 _ w1015 _ TRUE] -> w48
      event Timeout; "Sub Dir 1", "Sub Dir 2": Value Change {
        n30 = event-data() -> ()  [unwired: 1 in, 1 out]
        n31 = Unbundle(w130) -> ("Trajectory Data"=w119:T12, "Updated Waypoints"=w128:cluster{"x":dbl, "y":dbl, "th":dbl}[], "Cluster"=w129:T24)  [unwired: 1 out]
        n32 = List Folder(path=w126) -> (folder names=w133:string[], error out=w122:errorcluster)  [unwired: 3 in, 2 out]
        n33 = Index Array(array=w133, index="Sub Dir 1") -> (element=w134:string)
        n34 = Array Size(array=w133) -> (size(s)=w131:i32)
        n35 = property on="Sub Dir 1" class="Ring (strict)"("Strings []"=w133) -> ()  [unwired: 2 in, 2 out]
        n36 = case shown="1, Default" w131 {
          tunnel: w126 -> [w148 w151]
          tunnel: [w148 w150] -> w135
          tunnel: w134 -> [w147 w149]
          tunnel: [w147 w149] -> w115
          frame 0 {
          }
          frame 1, Default {
            n37 = Build Path(base path=w151, name or relative path=w149) -> (appended path=w150:path)
          }
        }
        n38 = List Folder(path=w135, error in=w122) -> (folder names=w132:string[], error out=w121:errorcluster)  [unwired: 2 in, 2 out]
        n39 = Array Size(array=w132) -> (size(s)=w136:i32)
        n40 = Index Array(array=w132, index="Sub Dir 2") -> (element=w140:string)
        n41 = property on="Sub Dir 2" class="Ring (strict)"("Strings []"=w132) -> ()  [unwired: 2 in, 2 out]
        n42 = call <vilib>:"Clear Errors.vi"("error in (no error)"=w121) -> ()  [unwired: 5 in, 2 out]
        n43 = Not Equal To 0?(x=w136) -> (x != 0?=w139:bool)
        n44 = case shown="False" w139 {
          tunnel: w135 -> [w154 w158]
          tunnel: [w154 w157] -> w125
          tunnel: w140 -> [w152 w155]
          tunnel: [2 0] -> w138
          tunnel: [w152 w155] -> w116
          frame False {
          }
          frame True {
            n45 = Build Path(base path=w158, name or relative path=w155) -> (appended path=w157:path)
          }
        }
        n46 = property on="Sub Dir 2" class="Ring (strict)"("DisabledEnum"=w138) -> ()  [unwired: 2 in, 2 out]
        n47 = Bundle(w115, w116) -> (→"folder names":cluster{string, string})  [unwired: 1 in]
        n48 = call <vilib>:"Recursive File List.vi"("Folder Path"=w125) -> ("error out"=w143:errorcluster, "All Files in Dir"=w146:path[])  [unwired: 6 in, 3 out]
        n49 = for {
          tunnel: w146 -> [w161] mode=indexing
          tunnel: [w171] -> w145 mode=indexing
          tunnel: w129 -> [w166]
          tunnel: w144 -> [w165]
          tunnel: w143 -> [_]
          tunnel: w119 -> [w160]
          tunnel: w118 -> [w159]
          n50 = Read from Binary File(5:"", 11:w161) -> (2:w169:string, 3:w168:refnum<file>)  [unwired: 4 in, 2 out]
          n51 = Strip Path(path=w161) -> (name=w162:string)  [unwired: 1 out]
          n52 = case shown="\"2.9\"" w169 {
            tunnel: [w173 w187 w201 w215 w229 w246 w265] -> w164
            tunnel: [w173 w186 w200 w214 w228 w245 w264] -> w163
            tunnel: w168 -> [w172 w185 w199 w213 w227 w244 w263]
            tunnel: [w172 w181 w195 w209 w223 w232 w248] -> w167
            tunnel: w166 -> [_ _ _ w202 w217 w235 w254]
            tunnel: w165 -> [_ w180 w194 w208 w222 w240 w259]
            tunnel: w160 -> [_ _ _ _ w216 w234 w253]
            tunnel: w159 -> [_ _ _ _ _ w231 w251]
            tunnel: [_ _ _ _ _ w230 w250] -> _
            frame Default {
              w173 = "?"
            }
            frame "2.0", "2.1" {
              n53 = Read from Binary File(5:T17 {"Velocity"=0.0, "Sample Time"=0.0, "Accel"=0.0}, 11:w185) -> (3:w184:refnum<file>)  [unwired: 4 in, 3 out]
              n54 = Read from Binary File(5:cluster{"x":dbl, "y":dbl, "th":dbl}[] [] ("Points"), 11:w184) -> (3:w183:refnum<file>)  [unwired: 4 in, 3 out]
              n55 = Read from Binary File(5:T12 [] ("Trajectory Data"), 11:w183) -> (3:w182:refnum<file>)  [unwired: 4 in, 3 out]
              n56 = Read from Binary File(5:w180, 11:w182) -> (2:w175:cluster{"Time (s)":dbl, "Distance (ft)":dbl}, 3:w181:refnum<file>)  [unwired: 4 in, 2 out]
              n57 = Unbundle(w175) -> ("Time (s)"=w179:dbl, "Distance (ft)"=w178:dbl)
              n58 = Format Into String(w179) -> (resulting string=w187:string)  [unwired: 3 in, 1 out]
              n59 = Format Into String(w178) -> (resulting string=w186:string)  [unwired: 3 in, 1 out]
            }
            frame "2.3" {
              n60 = Read from Binary File(5:T18 {"Sample Period (s)"=0.0, "Limits"={"Velocity (fps)"=0.0, "Acceleration (fps^2)"=0.0, "Jerk (fps^3)"=0.0}, "Conditions"={"vInitial (fps)"=0.0, "vFinal (fps)"=0.0}}, 11:w199) -> (3:w198:refnum<file>)  [unwired: 4 in, 3 out]
              n61 = Read from Binary File(5:cluster{"x":dbl, "y":dbl, "th":dbl}[] [] ("Points"), 11:w198) -> (3:w197:refnum<file>)  [unwired: 4 in, 3 out]
              n62 = Read from Binary File(5:T12 [] ("Trajectory Data"), 11:w197) -> (3:w196:refnum<file>)  [unwired: 4 in, 3 out]
              n63 = Read from Binary File(5:w194, 11:w196) -> (2:w189:cluster{"Time (s)":dbl, "Distance (ft)":dbl}, 3:w195:refnum<file>)  [unwired: 4 in, 2 out]
              n64 = Unbundle(w189) -> ("Time (s)"=w193:dbl, "Distance (ft)"=w192:dbl)
              n65 = Format Into String(w193) -> (resulting string=w201:string)  [unwired: 3 in, 1 out]
              n66 = Format Into String(w192) -> (resulting string=w200:string)  [unwired: 3 in, 1 out]
            }
            frame "2.5" {
              n67 = Read from Binary File(5:w202, 11:w213) -> (3:w212:refnum<file>)  [unwired: 4 in, 3 out]
              n68 = Read from Binary File(5:cluster{"x":dbl, "y":dbl, "th":dbl}[] [] ("Points"), 11:w212) -> (3:w211:refnum<file>)  [unwired: 4 in, 3 out]
              n69 = Read from Binary File(5:T12 [] ("Trajectory Data"), 11:w211) -> (3:w210:refnum<file>)  [unwired: 4 in, 3 out]
              n70 = Read from Binary File(5:w208, 11:w210) -> (2:w203:cluster{"Time (s)":dbl, "Distance (ft)":dbl}, 3:w209:refnum<file>)  [unwired: 4 in, 2 out]
              n71 = Unbundle(w203) -> ("Time (s)"=w207:dbl, "Distance (ft)"=w206:dbl)
              n72 = Format Into String(w207) -> (resulting string=w215:string)  [unwired: 3 in, 1 out]
              n73 = Format Into String(w206) -> (resulting string=w214:string)  [unwired: 3 in, 1 out]
            }
            frame "2.6", "2.7" {
              n74 = Read from Binary File(5:w217, 11:w227) -> (3:w226:refnum<file>)  [unwired: 4 in, 3 out]
              n75 = Read from Binary File(5:cluster{"x":dbl, "y":dbl, "th":dbl}[] [] ("Points"), 11:w226) -> (3:w225:refnum<file>)  [unwired: 4 in, 3 out]
              n76 = Read from Binary File(5:w216, 11:w225) -> (3:w224:refnum<file>)  [unwired: 4 in, 3 out]
              n77 = Read from Binary File(5:w222, 11:w224) -> (2:w218:cluster{"Time (s)":dbl, "Distance (ft)":dbl}, 3:w223:refnum<file>)  [unwired: 4 in, 2 out]
              n78 = Unbundle(w218) -> ("Time (s)"=w221:dbl, "Distance (ft)"=w220:dbl)
              n79 = Format Into String(w221) -> (resulting string=w229:string)  [unwired: 3 in, 1 out]
              n80 = Format Into String(w220) -> (resulting string=w228:string)  [unwired: 3 in, 1 out]
            }
            frame "2.8" {
              n81 = Read from Binary File(5:w235, 11:w244) -> (3:w243:refnum<file>)  [unwired: 4 in, 3 out]
              n82 = Read from Binary File(5:cluster{"x":dbl, "y":dbl, "th":dbl}[] [] ("Points"), 11:w243) -> (3:w242:refnum<file>)  [unwired: 4 in, 3 out]
              n83 = Read from Binary File(5:w234, 11:w242) -> (3:w241:refnum<file>)  [unwired: 4 in, 3 out]
              n84 = Read from Binary File(5:w240, 11:w241) -> (2:w236:cluster{"Time (s)":dbl, "Distance (ft)":dbl}, 3:w233:refnum<file>)  [unwired: 4 in, 2 out]
              n85 = Read from Binary File(5:w231, 11:w233) -> (0:w230:errorcluster, 3:w232:refnum<file>)  [unwired: 4 in, 2 out]
              n86 = Unbundle(w236) -> ("Time (s)"=w239:dbl, "Distance (ft)"=w238:dbl)
              n87 = Format Into String(w239) -> (resulting string=w246:string)  [unwired: 3 in, 1 out]
              n88 = Format Into String(w238) -> (resulting string=w245:string)  [unwired: 3 in, 1 out]
            }
            frame "2.9" {
              n89 = Read from Binary File(5:w254, 11:w263) -> (3:w262:refnum<file>)  [unwired: 4 in, 3 out]
              n90 = Read from Binary File(5:cluster{"x":dbl, "y":dbl, "th":dbl}[] [] ("Points"), 11:w262) -> (3:w261:refnum<file>)  [unwired: 4 in, 3 out]
              n91 = Read from Binary File(5:w253, 11:w261) -> (3:w260:refnum<file>)  [unwired: 4 in, 3 out]
              n92 = Read from Binary File(5:w259, 11:w260) -> (2:w255:cluster{"Time (s)":dbl, "Distance (ft)":dbl}, 3:w252:refnum<file>)  [unwired: 4 in, 2 out]
              n93 = Read from Binary File(5:w251, 11:w252) -> (0:w250:errorcluster, 3:w249:refnum<file>)  [unwired: 4 in, 2 out]
              n94 = Read from Binary File(5:T1 {"Path Backwards"=FALSE, "Robot Backwards"=FALSE} ("Cluster"), 11:w249) -> (3:w248:refnum<file>)  [unwired: 4 in, 3 out]
              n95 = Unbundle(w255) -> ("Time (s)"=w258:dbl, "Distance (ft)"=w257:dbl)
              n96 = Format Into String(w258) -> (resulting string=w265:string)  [unwired: 3 in, 1 out]
              n97 = Format Into String(w257) -> (resulting string=w264:string)  [unwired: 3 in, 1 out]
            }
          }
          n98 = Close File(refnum=w167) -> ()  [unwired: 1 in, 2 out]
          n99 = Build Array(w162, w164, w163) -> (w171:string[])
        }
        n100 = property on="Open" class="MCListbox (strict)"("ItemNames"=w145) -> ()  [unwired: 2 in, 2 out]
        n101 = First Call?() -> (First Call?: T/F=w117:bool)
      }
      event "New": Value Change {
        # "Use Initial Location"
        n102 = event-data() -> ()  [unwired: 1 in, 1 out]
        n103 = Unbundle(w271) -> ("Updated Waypoints"=w270:cluster{"x":dbl, "y":dbl, "th":dbl}[])  [unwired: 3 out]
        n104 = local write "Conditions"(T9 {"vInitial (fps)"=0.0, "vFinal (fps)"=0.0} ("Conditions")) -> ()
      }
      event "Append": Value Change {
        n105 = event-data() -> ()  [unwired: 1 in, 1 out]
        n106 = local read "Limits"() -> (w286:T8)
        n107 = Unbundle(w281) -> ("Updated Waypoints"=w280:cluster{"x":dbl, "y":dbl, "th":dbl}[])  [unwired: 3 out]
        n108 = local read "Conditions"() -> (w290:T9)
        n109 = Unbundle(w286) -> ("Velocity (fps)"=w285:dbl, "Accel (fps^2)"=w284:dbl)  [unwired: 1 out]
        n110 = Delete From Array(array=w280) -> (deleted portion=w292:cluster{"x":dbl, "y":dbl, "th":dbl})  [unwired: 2 in, 1 out]
        n111 = Divide(x=w285, y=w284) -> (x/y=w294:dbl)
        n112 = Build Array(w292) -> (w291:cluster{"x":dbl, "y":dbl, "th":dbl}[])
        n113 = Unbundle(w290) -> ("vFinal (fps)"=w289:dbl)  [unwired: 1 out]
        n114 = call "Add First Point.vi"("Accel (f/s^2)"=w284, "Time (s)"=w294, "Initial Points"=w291) -> ("Points"=w293:cluster{"x":dbl, "y":dbl, "th":dbl}[])  [unwired: 8 in]
        n115 = Bundle("vFinal (fps)"=w289, 0.0) -> (w288:cluster{"vFinal (fps)":dbl, dbl})  [unwired: 1 in]
        n116 = local write "Conditions"(w288) -> ()
      }
      event "Play": Value Change {
        n117 = event-data() -> ()  [unwired: 1 in, 1 out]
        n118 = Unbundle(w300) -> ("Updated Waypoints"=w299:cluster{"x":dbl, "y":dbl, "th":dbl}[])  [unwired: 3 out]
        n119 = Tick Count (ms)() -> (millisecond timer value=w301:u32)
        n120 = Generate User Event(user event=w303, event data cluster=w301) -> ()  [unwired: 2 in, 2 out]
      }
      event "Save": Value Change {
        n121 = event-data() -> ()  [unwired: 1 in, 1 out]
        n122 = Unbundle(w325) -> ("Trajectory Data"=w310:T12, "Updated Waypoints"=w322:cluster{"x":dbl, "y":dbl, "th":dbl}[], "Cluster"=w324:T24)  [unwired: 1 out]
        n123 = case shown="False" "Zero Vel" {
          tunnel: w310 -> [w335 w337]
          tunnel: [w335 w336] -> w309
          frame False {
          }
          frame True {
            n124 = for {
              tunnel: w337 -> [w340] mode=indexing
              tunnel: [w338] -> w336 mode=indexing
              n125 = Unbundle(w340) -> ("Traj Vel Points"=w341:cluster{"V":dbl, "th":dbl}[])  [unwired: 5 out]
              n126 = for {
                tunnel: w341 -> [w344] mode=indexing
                tunnel: [w342] -> w339 mode=indexing
                n127 = Unbundle(w344) -> ()  [unwired: 2 out]
                n128 = Bundle(cluster=w344, "V"=0.0) -> (w342:cluster{"V":dbl, "th":dbl})  [unwired: 1 in]
              }
              n129 = Bundle(cluster=w340, "Traj Vel Points"=w339) -> (w338:T25)  [unwired: 5 in]
            }
          }
        }
        n130 = local read "folder names"() -> (w316:cluster{"name":string, "name":string})
        n131 = Unbundle(w316) -> ("name"=w314:string, "name"=w313:string)
        n132 = call "Append String To Path.vi"("name"=w314, "path in"=w315) -> ("appended path out"=w312:path)  [unwired: 9 in]
        n133 = call "Append String To Path.vi"("name"=w313, "path in"=w312) -> ("appended path out"=w311:path)  [unwired: 9 in]
        n134 = Build Path(base path=w311, name or relative path="Filename") -> (appended path=w330:path)
        n135 = Write to Binary File(file (use dialog)=w330, data="2.9") -> (refnum out=w329:refnum<file>)  [unwired: 4 in, 2 out]
        n136 = Write to Binary File(file (use dialog)=w329, data=w324) -> (refnum out=w333:refnum<file>)  [unwired: 4 in, 2 out]
        n137 = Write to Binary File(file (use dialog)=w333, data=w322) -> (refnum out=w332:refnum<file>)  [unwired: 4 in, 2 out]
        n138 = Write to Binary File(file (use dialog)=w332, data=w309) -> (refnum out=w331:refnum<file>)  [unwired: 4 in, 2 out]
        n139 = Write to Binary File(file (use dialog)=w331, data=w318) -> (refnum out=w326:refnum<file>)  [unwired: 4 in, 2 out]
        n140 = Write to Binary File(file (use dialog)=w326, data=w317) -> (refnum out=w307:refnum<file>)  [unwired: 4 in, 2 out]
        n141 = Bundle("Trajectory Data"=w309, "Updated Waypoints"=w322, "Cluster"=w324, w317) -> (w327:T26)  [unwired: 1 in]
        n142 = Write to Binary File(file (use dialog)=w307, data="Cluster") -> (refnum out=w306:refnum<file>)  [unwired: 4 in, 2 out]
        n143 = Close File(refnum=w306) -> ()  [unwired: 1 in, 2 out]
      }
      event "Open Command": Value Change {
        n144 = event-data() -> ()  [unwired: 1 in, 1 out]
        n145 = Unbundle(w354) -> ("Updated Waypoints"=w353:cluster{"x":dbl, "y":dbl, "th":dbl}[])  [unwired: 3 out]
        n146 = call "Open Command Panel.vi"("Commands"=w352, "Tag"="Command Sequence") -> ("Found"=w349:bool)  [unwired: 9 in]
        n147 = Select(t="Command Sequence", s=w349, f="") -> (s? t:f=w346:string)
        n148 = Bundle(cluster=w350, "Filename"=w346) -> (w351:T15)  [unwired: 2 in]
      }
      event "Directory": Value Change {
        n149 = event-data() -> ()  [unwired: 1 in, 1 out]
        n150 = Unbundle(w371) -> ("Updated Waypoints"=w370:cluster{"x":dbl, "y":dbl, "th":dbl}[])  [unwired: 3 out]
        n151 = call "File Dialog"("start path"=w364, "prompt"="Path Folder", "button label"="Select") -> ("selected path"=w363:path, "error out"=w365:errorcluster)  [unwired: 9 in, 2 out]
        n152 = Select(t=w364, s=w365, f=w363) -> (s? t:f=w362:path)
        n153 = Format Into String(format string=w367, w362) -> (resulting string=w368:string)  [unwired: 2 in, 1 out]
        n154 = property class="VI"("Front Panel.Title"=w368) -> ()  [unwired: 2 in, 2 out]
      }
      event "Open": Double Click {
        # "Need the Waypoints in the file TODO"
        n155 = event-data() -> ("Row"=w407:i32)  [unwired: 1 in]
        n156 = property on="Open" class="MCListbox (strict)"() -> ("ItemNames"=w408:string[][])  [unwired: 2 in, 2 out]
        n157 = local read "folder names"() -> (w386:cluster{"name":string, "name":string})
        n158 = Index Array(array=w408, index (row)=w407, index (col)=0 ("disabled index (col)")) -> (element=w398:string)
        n159 = Unbundle(w386) -> ("name"=w375:string, "name"=w378:string)
        n160 = call "Append String To Path.vi"("name"=w375, "path in"=w377) -> ("appended path out"=w376:path)  [unwired: 9 in]
        n161 = call "Append String To Path.vi"("name"=w378, "path in"=w376) -> ("appended path out"=w385:path)  [unwired: 9 in]
        n162 = Build Path(base path=w385, name or relative path=w398) -> (appended path=w399:path)
        n163 = local write "Filename"(w398) -> ()
        n164 = Unbundle(w389) -> ("Trajectory Data"=w382:T12, "Cluster"=w388:T24)  [unwired: 2 out]
        n165 = Read from Binary File(5:"", 11:w399) -> (2:w404:string, 3:w403:refnum<file>)  [unwired: 4 in, 2 out]
        n166 = case shown="\"2.9\"" w404 {
          tunnel: w403 -> [w411 w428 w444 w460 w480 w497 w516 w536 w559]
          tunnel: w388 -> [_ _ _ _ _ w486 w506 w526 w549]
          tunnel: w402 -> [_ w426 w442 w458 w478 w495 w514 w534 w557]
          tunnel: [_ w425 w441 w457 w477 w494 w513 w533 w556] -> w390
          tunnel: w382 -> [_ w424 w440 w456 w476 w493 w512 w532 w555]
          tunnel: w400 -> [_ w422 w438 w454 w474 w491 w510 w530 w553]
          tunnel: [w411 w420 w436 w452 w472 w489 w501 w521 w540] -> w401
          tunnel: [_ w418 w435 w451 w471 w488 w508 w528 w551] -> w397
          tunnel: [_ w417 w434 w450 w470 w487 w507 w527 w550] -> w396
          tunnel: [_ _ w433 w449 w469 w485 w505 w525 w548] -> w395
          tunnel: [T13 {"Angular \nAccelerations"=[], "Override Limits?"=[]} ("Angular Accelerations") T13 {"Angular \nAccelerations"=[], "Override Limits?"=[]} ("Angular Accelerations") T13 {"Angular \nAccelerations"=[], "Override Limits?"=[]} ("Angular Accelerations") T13 {"Angular \nAccelerations"=[], "Override Limits?"=[]} ("Angular Accelerations") w463 w484 w504 w524 w547] -> w394
          tunnel: [T12 [] ("Trajectory Data") w412 w430 w446 w462 w483 w503 w523 w546] -> w391
          tunnel: [_ _ _ _ _ _ w500 _ _] -> _
          tunnel: w381 -> [_ _ _ _ _ _ _ w520 w544]
          tunnel: [_ _ _ _ _ _ _ w519 w543] -> w380
          tunnel: [_ _ _ _ _ _ _ w518 w542] -> _
          tunnel: [_ _ _ _ _ _ _ _ w538] -> w374
          frame "False", Default {
          }
          frame "2.0", "2.1" {
            n167 = Read from Binary File(5:T17 {"Velocity"=0.0, "Sample Time"=0.0, "Accel"=0.0}, 11:w428) -> (2:w429:T17, 3:w427:refnum<file>)  [unwired: 4 in, 2 out]
            n168 = Read from Binary File(5:w426, 11:w427) -> (2:w425:cluster{"x":dbl, "y":dbl, "th":dbl}[], 3:w423:refnum<file>)  [unwired: 4 in, 2 out]
            n169 = Unbundle(w429) -> ("Velocity"=w416:dbl, "Sample Time"=w418:dbl, "Accel"=w415:dbl)
            n170 = Read from Binary File(5:w424, 11:w423) -> (2:w412:T12, 3:w421:refnum<file>)  [unwired: 4 in, 2 out]
            n171 = Read from Binary File(5:w422, 11:w421) -> (3:w420:refnum<file>)  [unwired: 4 in, 3 out]
            n172 = Bundle("Velocity"=w416, "Accel"=w415, "Accel"=1000.0) -> (w417:T27)  [unwired: 1 in]
          }
          frame "2.3" {
            n173 = Read from Binary File(5:T18 {"Sample Period (s)"=0.0, "Limits"={"Velocity (fps)"=0.0, "Acceleration (fps^2)"=0.0, "Jerk (fps^3)"=0.0}, "Conditions"={"vInitial (fps)"=0.0, "vFinal (fps)"=0.0}}, 11:w444) -> (2:w445:T18, 3:w443:refnum<file>)  [unwired: 4 in, 2 out]
            n174 = Unbundle(w445) -> ("Sample Period (s)"=w435:dbl, "Limits"=w434:T28, "Conditions"=w433:T9)
            n175 = Read from Binary File(5:w442, 11:w443) -> (2:w441:cluster{"x":dbl, "y":dbl, "th":dbl}[], 3:w439:refnum<file>)  [unwired: 4 in, 2 out]
            n176 = Read from Binary File(5:w440, 11:w439) -> (2:w430:T12, 3:w437:refnum<file>)  [unwired: 4 in, 2 out]
            n177 = Read from Binary File(5:w438, 11:w437) -> (3:w436:refnum<file>)  [unwired: 4 in, 3 out]
          }
          frame "2.4" {
            n178 = Read from Binary File(5:T18 {"Sample Period (s)"=0.0, "Limits"={"Velocity (fps)"=0.0, "Acceleration (fps^2)"=0.0, "Jerk (fps^3)"=0.0}, "Conditions"={"vInitial (fps)"=0.0, "vFinal (fps)"=0.0}}, 11:w460) -> (2:w461:T18, 3:w459:refnum<file>)  [unwired: 4 in, 2 out]
            n179 = Unbundle(w461) -> ("Sample Period (s)"=w451:dbl, "Limits"=w450:T28, "Conditions"=w449:T9)
            n180 = Read from Binary File(5:w458, 11:w459) -> (2:w457:cluster{"x":dbl, "y":dbl, "th":dbl}[], 3:w455:refnum<file>)  [unwired: 4 in, 2 out]
            n181 = Read from Binary File(5:w456, 11:w455) -> (2:w446:T12, 3:w453:refnum<file>)  [unwired: 4 in, 2 out]
            n182 = Read from Binary File(5:w454, 11:w453) -> (3:w452:refnum<file>)  [unwired: 4 in, 3 out]
          }
          frame "2.5" {
            n183 = Read from Binary File(5:T19 {"Sample Period (s)"=0.0, "Limits"={"Velocity (fps)"=0.0, "Acceleration (fps^2)"=0.0, "Jerk (fps^3)"=0.0}, "Conditions"={"vInitial (fps)"=0.0, "vFinal (fps)"=0.0}, "Min Rads"=[20.0, 20.0, 20.0, 20.0, 20.0]}, 11:w480) -> (2:w481:T19, 3:w479:refnum<file>)  [unwired: 4 in, 2 out]
            n184 = Unbundle(w481) -> ("Sample Period (s)"=w471:dbl, "Limits"=w470:T28, "Conditions"=w469:T9, "Min Rads"=w465:dbl[])
            n185 = Array Size(array=w465) -> (size(s)=w466:i32)
            n186 = for {
              N: w466 -> [_]
              tunnel: [TRUE] -> w464 mode=indexing
            }
            n187 = Read from Binary File(5:w478, 11:w479) -> (2:w477:cluster{"x":dbl, "y":dbl, "th":dbl}[], 3:w475:refnum<file>)  [unwired: 4 in, 2 out]
            n188 = Read from Binary File(5:w476, 11:w475) -> (2:w462:T12, 3:w473:refnum<file>)  [unwired: 4 in, 2 out]
            n189 = Bundle(cluster=T13 {"Angular \nAccelerations"=[], "Override Limits?"=[]} ("Angular Accelerations"), "Angular \nAccelerations"=w465, "Override Limits?"=w464) -> (w463:T13)
            n190 = Read from Binary File(5:w474, 11:w473) -> (3:w472:refnum<file>)  [unwired: 4 in, 3 out]
          }
          frame "2.6" {
            n191 = Read from Binary File(5:w486, 11:w497) -> (2:w498:T24, 3:w496:refnum<file>)  [unwired: 4 in, 2 out]
            n192 = Unbundle(w498) -> ("Sample Period (s)"=w488:dbl, "Limits"=w487:T8, "Conditions"=w485:T9, "Acceleration Overrides"=w484:T7)
            n193 = Read from Binary File(5:w495, 11:w496) -> (2:w494:cluster{"x":dbl, "y":dbl, "th":dbl}[], 3:w492:refnum<file>)  [unwired: 4 in, 2 out]
            n194 = Read from Binary File(5:w493, 11:w492) -> (2:w483:T12, 3:w490:refnum<file>)  [unwired: 4 in, 2 out]
            n195 = Read from Binary File(5:w491, 11:w490) -> (3:w489:refnum<file>)  [unwired: 4 in, 3 out]
          }
          frame "2.7" {
            n196 = Read from Binary File(5:w506, 11:w516) -> (2:w517:T24, 3:w515:refnum<file>)  [unwired: 4 in, 2 out]
            n197 = Unbundle(w517) -> ("Sample Period (s)"=w508:dbl, "Limits"=w507:T8, "Conditions"=w505:T9, "Acceleration Overrides"=w504:T7)
            n198 = Read from Binary File(5:w514, 11:w515) -> (2:w513:cluster{"x":dbl, "y":dbl, "th":dbl}[], 3:w511:refnum<file>)  [unwired: 4 in, 2 out]
            n199 = Read from Binary File(5:w512, 11:w511) -> (2:w503:T12, 3:w509:refnum<file>)  [unwired: 4 in, 2 out]
            n200 = Read from Binary File(5:w510, 11:w509) -> (3:w502:refnum<file>)  [unwired: 4 in, 3 out]
            n201 = Read from Binary File(5:T21 [] ("Commands"), 11:w502) -> (2:w500:T21, 3:w501:refnum<file>)  [unwired: 4 in, 2 out]
          }
          frame "2.8" {
            n202 = Read from Binary File(5:w526, 11:w536) -> (2:w537:T24, 3:w535:refnum<file>)  [unwired: 4 in, 2 out]
            n203 = Unbundle(w537) -> ("Sample Period (s)"=w528:dbl, "Limits"=w527:T8, "Conditions"=w525:T9, "Acceleration Overrides"=w524:T7)
            n204 = Read from Binary File(5:w534, 11:w535) -> (2:w533:cluster{"x":dbl, "y":dbl, "th":dbl}[], 3:w531:refnum<file>)  [unwired: 4 in, 2 out]
            n205 = Read from Binary File(5:w532, 11:w531) -> (2:w523:T12, 3:w529:refnum<file>)  [unwired: 4 in, 2 out]
            n206 = Read from Binary File(5:w530, 11:w529) -> (3:w522:refnum<file>)  [unwired: 4 in, 3 out]
            n207 = Read from Binary File(5:w520, 11:w522) -> (0:w518:errorcluster, 2:w519:cluster{"Time (s)":dbl, T3, bool}[], 3:w521:refnum<file>)  [unwired: 4 in, 1 out]
          }
          frame "2.9" {
            n208 = Read from Binary File(5:w549, 11:w559) -> (2:w560:T24, 3:w558:refnum<file>)  [unwired: 4 in, 2 out]
            n209 = Unbundle(w560) -> ("Sample Period (s)"=w551:dbl, "Limits"=w550:T8, "Conditions"=w548:T9, "Acceleration Overrides"=w547:T7)
            n210 = Read from Binary File(5:w557, 11:w558) -> (2:w556:cluster{"x":dbl, "y":dbl, "th":dbl}[], 3:w554:refnum<file>)  [unwired: 4 in, 2 out]
            n211 = Read from Binary File(5:w555, 11:w554) -> (2:w546:T12, 3:w552:refnum<file>)  [unwired: 4 in, 2 out]
            n212 = Read from Binary File(5:w553, 11:w552) -> (3:w545:refnum<file>)  [unwired: 4 in, 3 out]
            n213 = Read from Binary File(5:w544, 11:w545) -> (0:w542:errorcluster, 2:w543:cluster{"Time (s)":dbl, T3, bool}[], 3:w541:refnum<file>)  [unwired: 4 in, 1 out]
            n214 = Read from Binary File(5:T1 {"Path Backwards"=FALSE, "Robot Backwards"=FALSE} ("Cluster"), 11:w541) -> (2:w538:T1, 3:w540:refnum<file>)  [unwired: 4 in, 2 out]
          }
        }
        n215 = Close File(refnum=w401) -> ()  [unwired: 1 in, 2 out]
        n216 = Bundle("Sample Period (s)"=w397, "Limits"=w396, "Conditions"=w395, "Acceleration Overrides"=w394) -> (w393:T24)  [unwired: 1 in]
        n217 = local write "Acceleration Overrides"(w394) -> ()
        n218 = local write "Cluster"(w374) -> ()
        n219 = local write "Sample Period (s)"(w397) -> ()
        n220 = local write "Limits"(w396) -> ()
        n221 = local write "Conditions"(w395) -> ()
        n222 = Bundle("Trajectory Data"=w391, "Points"=w390, w393, w380) -> (w392:T29)  [unwired: 1 in]
      }
      event "Picture": Mouse Down {
        n223 = event-data() -> ("Coords"=w575:T30, "Button"=w577:u16, "Mods"=w576:cluster{"Double Click":bool, "Menu Key":bool}, "PlatMods"=w572:T31)  [unwired: 1 in]
        n224 = Unbundle(w569) -> ("Updated Waypoints"=w568:cluster{"x":dbl, "y":dbl, "th":dbl}[])  [unwired: 3 out]
        n225 = Unbundle(w565) -> ("Drag Object"=w564:cluster{"Index":i32, "x":dbl, "y":dbl})  [unwired: 2 out]
        n226 = case shown="1" w577 {
          tunnel: w576 -> [_ _ w589]
          tunnel: w575 -> [_ _ w594]
          tunnel: w568 -> [w581 w585 w595]
          tunnel: [w581 w585 w599] -> w574
          tunnel: w573 -> [_ _ w596]
          tunnel: w564 -> [w579 w582 w590]
          tunnel: [w578 w584 w591] -> w566
          tunnel: w572 -> [_ _ w587]
          frame 0, Default {
            # "middle mouse?"
            n227 = Bundle(cluster=w579, "Index"=-1) -> (w578:cluster{"Index":i32, "x":dbl, "y":dbl})  [unwired: 2 in]
          }
          frame 2 {
            # "Right Button"
            n228 = Bundle(cluster=w582, "Index"=-1) -> (w584:cluster{"Index":i32, "x":dbl, "y":dbl})  [unwired: 2 in]
          }
          frame 1 {
            # "Left Button"
            n229 = Unbundle By Name(w589) -> ("Double Click"=w588:bool)
            n230 = property on="Picture" class="Pict"() -> ("Position"=w598:T10, "Draw Area Size"=w597:T32)  [unwired: 2 in, 2 out]
            n231 = Unbundle By Name(w587) -> ("Shift"=w586:bool)
            n232 = call "Point Test Shapes.vi"("Coords"=w594, "Points"=w595, "Picture in"=w596) -> ("Pt Test Results"=w593:enum16{"Miss", "Rect Hit", "Arrow Hit"}, "Results"=w592:T14)  [unwired: 7 in]
            n233 = case shown="\"Miss\", Default" w593 {
              tunnel: w588 -> [_ _ w642]
              tunnel: w595 -> [w603 w631 w636]
              tunnel: w592 -> [_ w629 w643]
              tunnel: [w606 w632 w635] -> w599
              tunnel: w594 -> [w607 _ _]
              tunnel: w598 -> [w605 _ _]
              tunnel: w597 -> [w604 _ _]
              tunnel: [w601 w624 w639] -> w591
              tunnel: w590 -> [w600 _ w640]
              tunnel: w586 -> [w602 _ w637]
              frame "Miss", Default {
                n234 = case shown="True" w602 {
                  tunnel: w607 -> [w619 _]
                  tunnel: [w616 w623] -> w606
                  tunnel: w605 -> [w615 _]
                  tunnel: w604 -> [w614 _]
                  tunnel: w603 -> [w610 w623]
                  tunnel: [w609 w622] -> w601
                  tunnel: w600 -> [_ w620]
                  frame False {
                    n235 = call "Map to Feet.vi"("Draw Area Size"=w614, "Position"=w615, "Coords (px)"=w619) -> ("Point (ft)"=w613:cluster{dbl, dbl})  [unwired: 8 in]
                    n236 = Array Size(array=w610) -> (size(s)=w608:i32)
                    n237 = Unbundle(w613) -> (w612:dbl, w611:dbl)
                    n238 = Bundle(w612, w611, nan) -> (w617:cluster{dbl, dbl, dbl})  [unwired: 1 in]
                    n239 = Bundle(w608, w612, w611) -> (w609:cluster{i32, dbl, dbl})  [unwired: 1 in]
                    n240 = Build Array (concatenate)(w610, w617) -> (w616:cluster{"x":dbl, "y":dbl, "th":dbl}[])
                  }
                  frame True {
                    n241 = Bundle(cluster=w620, "Index"=-1) -> (w622:cluster{"Index":i32, "x":dbl, "y":dbl})  [unwired: 2 in]
                  }
                }
              }
              frame "Arrow Hit" {
                # "start tracking rotation"
                n242 = Unbundle(w629) -> ("Index"=w628:i32)  [unwired: 1 out]
                n243 = Index Array(array=w631, index=w628) -> (element=w630:cluster{"x":dbl, "y":dbl, "th":dbl})
                n244 = Unbundle(w630) -> ("x"=w627:dbl, "y"=w626:dbl, "th"=w634:dbl)
                n245 = Bundle(cluster=w630, "th"=w634) -> (w633:cluster{"x":dbl, "y":dbl, "th":dbl})  [unwired: 2 in]
                n246 = Bundle(-2, "x"=w627, "y"=w626) -> (w624:cluster{i32, "x":dbl, "y":dbl})  [unwired: 1 in]
                n247 = Replace Array Subset(array=w631, new element=w633) -> (w632:cluster{"x":dbl, "y":dbl, "th":dbl}[])  [unwired: 1 in]
              }
              frame "Rect Hit" {
                n248 = Unbundle(w643) -> ("Index"=w641:i32)  [unwired: 1 out]
                n249 = case shown="False" w637 {
                  tunnel: w642 -> [w647 _]
                  tunnel: w641 -> [w646 w650]
                  tunnel: [w645 -1 ("length")] -> w638
                  tunnel: w636 -> [w644 w653]
                  tunnel: [w644 w652] -> w635
                  frame False {
                    n250 = case shown="False" w647 {
                      tunnel: w646 -> [w648 _]
                      tunnel: [w648 -1] -> w645
                      frame False {
                      }
                      frame True {
                        # "TODO Toggle last pt"
                      }
                    }
                  }
                  frame True {
                    n251 = case shown="Default" w650 {
                      tunnel: w653 -> [w654 w658]
                      tunnel: w650 -> [_ w657]
                      tunnel: [w654 w655] -> w652
                      frame 0 {
                      }
                      frame Default {
                        n252 = Delete From Array(array=w658, length=1, index=w657) -> (array with subset deleted=w655:cluster{"x":dbl, "y":dbl, "th":dbl}[])  [unwired: 1 out]
                      }
                    }
                  }
                }
                n253 = Bundle(cluster=w640, "Index"=w638) -> (w639:cluster{"Index":i32, "x":dbl, "y":dbl})  [unwired: 2 in]
              }
            }
          }
        }
        n254 = Bundle(cluster=w565, "Drag Object"=w566) -> (w567:T15)  [unwired: 2 in]
      }
      event "Picture": Mouse Move; "Picture": Mouse Up {
        n255 = event-data() -> ("Type"=w676:T22, "Coords"=w678:T30)  [unwired: 1 in]
        n256 = Unbundle(w669) -> ("Updated Waypoints"=w668:cluster{"x":dbl, "y":dbl, "th":dbl}[])  [unwired: 3 out]
        n257 = Unbundle(w661) -> ("Drag Object"=w664:cluster{"Index":i32, "x":dbl, "y":dbl})  [unwired: 2 out]
        n258 = Unbundle(w664) -> ("Index"=w675:i32)  [unwired: 2 out]
        n259 = case shown="Default" w675 {
          selector: w675 -> [w688 _]
          tunnel: w678 -> [w697 w705]
          tunnel: [w695 w704] -> w666
          tunnel: [w692 w703] -> w677
          tunnel: w668 -> [w693 w703]
          tunnel: [w689 w702] -> w667
          tunnel: w664 -> [w680 w702]
          tunnel: w676 -> [w690 _]
          tunnel: "Snap to foot" -> [w685 _]
          tunnel: "Snap robot to baseline" -> [w686 _]
          tunnel: "Angle Limiter" -> [w687 _]
          tunnel: w660 -> [w679 w701]
          tunnel: w659 -> [_ w700]
          frame Default {
            # "Mouse up changes indes to break tracking,\notherwise update coords"
            n260 = property on="Picture" class="Pict"() -> ("Position"=w698:T10, "Draw Area Size"=w699:T32)  [unwired: 2 in, 2 out]
            n261 = Bundle("Snap robot to baseline"=w686, "Snap to foot"=w685, "Angle Limiter"=w687) -> (w684:T33)  [unwired: 1 in]
            n262 = call "Map to Feet.vi"("Draw Area Size"=w699, "Position"=w698, "Coords (px)"=w697) -> ("Point (ft)"=w696:cluster{dbl, dbl})  [unwired: 8 in]
            n263 = Equal?(x=lveventtype."Mouse Up" ("Type"), y=w690) -> (x = y?=w683:bool)
            n264 = call "Handle Pos and Rot.vi"("Mouse Up"=w683, "Picture in"=w679, "Option"=w684, "Coord (ft)"=w696, "Index"=w688, "Points in"=w693) -> ("Points out"=w692:cluster{"x":dbl, "y":dbl, "th":dbl}[])  [unwired: 5 in]
            n265 = Bundle(cluster=w680, "Index"=-1) -> (w681:cluster{"Index":i32, "x":dbl, "y":dbl})  [unwired: 2 in]
            n266 = Bundle(w688, "Pt Test Results"=enum16{"Miss", "Rect Hit", "Arrow Hit"}."Rect Hit") -> (w695:T34)  [unwired: 1 in]
            n267 = Select(t=w681, s=w683, f=w680) -> (s? t:f=w689:cluster{"Index":i32, "x":dbl, "y":dbl})
          }
          frame -1 {
            n268 = call "Point Test Shapes.vi"("Array"=w700, "Coords"=w705, "Points"=w703, "Picture in"=w701) -> ("Results"=w704:T14)  [unwired: 6 in, 1 out]
          }
        }
        n269 = Bundle(cluster=w661, "Drag Object"=w667, "Hover Object"=w666) -> (w665:T15)  [unwired: 1 in]
      }
      event "Time (s)", "Snap to foot", "Angle Limiter", "Snap robot to baseline", "Limits", "Sample Period (s)", "Center Flip", "Conditions", "Unjank", "Acceleration Overrides": Value Change {
        # "Changes to any of these control will run the diagram to update the preview"
        n270 = event-data() -> ("CtlRef"=w719:refnum<vi>)  [unwired: 1 in]
        n271 = control-ref of="Center Flip"() -> (w720:refnum<vi>)
        n272 = Equal?(x=w720, y=w719) -> (x = y?=w718:bool)
        n273 = Unbundle(w713) -> ("Updated Waypoints"=w712:cluster{"x":dbl, "y":dbl, "th":dbl}[])  [unwired: 3 out]
        n274 = case shown="True" "Unjank" {
          tunnel: w713 -> [_ w725]
          tunnel: "Turn Acceleration" -> [_ w723]
          tunnel: "Turn Deceleration" -> [_ w722]
          frame False {
          }
          frame True {
            n275 = call "Turn Smother.vi"("Ignore Deceleration"=w722, "Ignore Acceleration"=w723, "input cluster"=w725) -> ("Angular Accelerations"=w724:T13)
            n276 = local write "Acceleration Overrides"(w724) -> ()
          }
        }
        n277 = case shown="True" w718 {
          tunnel: w712 -> [w726 w728]
          tunnel: [w726 w727] -> w721
          frame False {
          }
          frame True {
            n278 = for {
              tunnel: w728 -> [w736] mode=indexing
              tunnel: [w729] -> w727 mode=indexing
              n279 = Unbundle(w736) -> ("x"=w735:dbl, "y"=w731:dbl, "th"=w730:dbl)
              n280 = Negate(x=w735) -> (-x=w734:dbl)
              n281 = Add(x=27.0 ("y"), y=w734) -> (x+y=w732:dbl)
              n282 = Bundle(w732, "y"=w731, "th"=w730) -> (w729:cluster{dbl, "y":dbl, "th":dbl})  [unwired: 1 in]
            }
          }
        }
      }
      event Key Down?; event type 5.0.x8000000b {
        n283 = event-data() -> ("VKey"=w750:T35)  [unwired: 1 in]
        n284 = local read "Snap robot to baseline"() -> (w757:bool)
        n285 = Unbundle(w744) -> ("Updated Waypoints"=w743:cluster{"x":dbl, "y":dbl, "th":dbl}[])  [unwired: 3 out]
        n286 = local read "Angle Limiter"() -> (w755:enum16{"90", "45", "15", "1"})
        n287 = local read "Snap to foot"() -> (w756:bool)
        n288 = Unbundle(w741) -> ("Hover Object"=w742:T14)  [unwired: 2 out]
        n289 = case shown="\"Down\"" w750 {
          tunnel: [cluster{dbl, dbl} {0.0, 0.0} ("Coord (ft)") cluster{dbl, dbl} {0.0, 0.1} ("Coord (ft)") cluster{dbl, dbl} {0.0, -0.1} ("Coord (ft)") cluster{dbl, dbl} {-0.1, 0.0} ("Coord (ft)") cluster{dbl, dbl} {0.1, 0.0} ("Coord (ft)")] -> w752
          tunnel: [_ w770 w772 w774 w776] -> w748
          tunnel: TRUE ("Delta") -> [_ w770 w772 w774 w776]
          frame Default {
          }
          frame "Up" {
          }
          frame "Down" {
          }
          frame "Left" {
          }
          frame "Right" {
          }
        }
        n290 = Unbundle(w742) -> ("Index"=w740:i32, "Pt Test Results"=w749:enum16{"Miss", "Rect Hit", "Arrow Hit"})
        n291 = Bundle("Snap robot to baseline"=w757, "Snap to foot"=w756, "Angle Limiter"=w755) -> (w754:T33)  [unwired: 1 in]
        n292 = case shown="\"Rect Hit\", Default" w749 {
          tunnel: [w760 w768] -> w758
          tunnel: w745 -> [_ w767]
          tunnel: w754 -> [_ w766]
          tunnel: w743 -> [w760 w765]
          tunnel: TRUE ("Delta") -> [_ w764]
          tunnel: w752 -> [_ w763]
          tunnel: w748 -> [_ w762]
          tunnel: [_ w762] -> w747
          tunnel: w740 -> [_ w761]
          frame "Miss" {
          }
          frame "Rect Hit", Default {
            n293 = call "Handle Pos and Rot.vi"("Delta"=w764, "Picture in"=w767, "Option"=w766, "Coord (ft)"=w763, "Index"=w761, "Points in"=w765) -> ("Points out"=w768:cluster{"x":dbl, "y":dbl, "th":dbl}[])  [unwired: 5 in]
          }
        }
        n294 = event-data("Discard?"=w747) -> ()  [unwired: 1 in, 1 out]
      }
      event User Event {
        n295 = event-data() -> ("Data"=w790:i32)  [unwired: 1 in]
        n296 = Unbundle(w783) -> ("Updated Waypoints"=w782:cluster{"x":dbl, "y":dbl, "th":dbl}[])  [unwired: 3 out]
        n297 = Tick Count (ms)() -> (millisecond timer value=w793:u32)
        n298 = Subtract(x=w793, y=w790) -> (x-y=w792:u32)
        n299 = Multiply(x=w792, y=0.001) -> (x*y=w789:dbl)
        n300 = local read "Duration (s)"() -> (w795:dbl)
        n301 = Quotient & Remainder(x=w789, y=0.02) -> (floor(x/y)=w787:dbl)  [unwired: 1 out]
        n302 = Multiply(x=0.02, y=w787) -> (x*y=w786:dbl)
        n303 = Less Or Equal?(x=w786, y=w795) -> (x <= y?=w796:bool)
        n304 = case shown="True" w796 {
          tunnel: w797 -> [_ w801]
          tunnel: w790 -> [_ w799]
          tunnel: w786 -> [_ w800]
          frame False {
          }
          frame True {
            n305 = local write "Time (s)"(w800) -> ()
            n306 = Generate User Event(user event=w801, event data cluster=w799) -> ()  [unwired: 2 in, 2 out]
          }
        }
        n307 = Wait (ms)(milliseconds to wait=u32 50) -> ()  [unwired: 1 out]
      }
      event "Tab Control": Value Change {
        n308 = event-data() -> ("NewVal"=w806:T6)  [unwired: 1 in]
        n309 = Unbundle(w809) -> ("Updated Waypoints"=w808:cluster{"x":dbl, "y":dbl, "th":dbl}[])  [unwired: 3 out]
        n310 = case shown="\"Command Sequencer\"" w806 {
          tunnel: [w812 w813] -> w805
          tunnel: w804 -> [w812 _]
          frame "Trajectory Settings", Default {
          }
          frame "Command Sequencer" {
            n311 = call "Find RT Projects.vi"() -> ("Targets"=w813:refnum<vi>[], "Project Names"=w814:string[])  [unwired: 10 in]
            n312 = property on="Projects" class="Ring (strict)"("Strings []"=w814) -> ()  [unwired: 2 in, 2 out]
          }
        }
      }
      event "Refresh": Value Change {
        # "Later make this load from file so it doesn't need to be recomputed so often"
        n313 = event-data() -> ()  [unwired: 1 in, 1 out]
        n314 = Unbundle(w828) -> ("Updated Waypoints"=w827:cluster{"x":dbl, "y":dbl, "th":dbl}[])  [unwired: 3 out]
        n315 = Index Array(array=w825, index="Projects") -> (element=w823:refnum<vi>)
        n316 = call "Find Command Names.vi"("TargetItem in"=w823) -> ("Paths"=w822:path[], "Command Info"=w821:T36)  [unwired: 9 in]
        n317 = call "Format Commands to Tree.vi"("Paths"=w822, "Command Info"=w821) -> ("2D Picture"=w820:picture, "Filtered Command Info Out"=w817:T2)  [unwired: 8 in]
        n318 = call "Resize Icons.vi"("Scale Factor"="Scale Factor", "Filtered Command Info Out"=w817) -> ("Filtered Command Info Out"=w816:T2)  [unwired: 9 in]
        n319 = Bundle("Filtered Command Info Out"=w816, "2D Picture"=w820) -> (w819:T5)  [unwired: 1 in]
        n320 = local write "Command Palette"(w820) -> ()
        n321 = local write "Cache"(w819) -> ()
      }
      event event #0x53 {
        n322 = event-data() -> ("AppRef"=w836:refnum<vi>, "VIName"=w838:string, "VIAppRef"=w834:refnum<vi>)  [unwired: 1 in, 1 out]
        n323 = Unbundle(w848) -> ("Updated Waypoints"=w847:cluster{"x":dbl, "y":dbl, "th":dbl}[])  [unwired: 3 out]
        n324 = Unbundle(w846) -> ("Filename"=w837:string)  [unwired: 2 out]
        n325 = property class="App"(reference=w836) -> ("App.Name"=w835:string)  [unwired: 1 in, 2 out]
        n326 = property class="App"(reference=w834) -> ("App.Name"=w833:string)  [unwired: 1 in, 2 out]
        n327 = Search and Replace String(input string=w837, search string=w838, replace string=w838) -> (number of replacements=w843:i32)  [unwired: 5 in, 3 out]
        n328 = call "Find Command with Tag.vi"("Command Tag"=w837, "Commands"=w832) -> ("Index"=w844:i32, "Found Command"=w845:cluster{"Time (s)":dbl, T3, bool}, "Found"=w841:bool)  [unwired: 7 in]
        n329 = Not Equal To 0?(x=w843) -> (x != 0?=w842:bool)
        n330 = And(x=w841, y=w842) -> (x .and. y?=w840:bool)
        n331 = case shown="True" w840 {
          tunnel: w845 -> [_ w860]
          tunnel: w844 -> [_ w866]
          tunnel: w832 -> [w852 w868]
          tunnel: [w852 w867] -> _
          tunnel: [_ FALSE] -> w839
          tunnel: w835 -> [_ _]
          tunnel: w833 -> [_ _]
          frame False {
          }
          frame True {
            n332 = Unbundle(w860) -> (w862:T3)  [unwired: 2 out]
            n333 = Unbundle(w862) -> ("Path"=w854:path)  [unwired: 6 out]
            n334 = call "Localize Path.vi"("Path"=w854) -> ("Local path"=w853:path)
            n335 = Open VI Reference(vi path=w853) -> (vi reference=w864:refnum<vi>)  [unwired: 5 in, 1 out]
            n336 = property class="VI"(reference=w864) -> (reference out=w857:refnum<vi>, "Panel"=w865:refnum<vi>)  [unwired: 1 in, 1 out]
            n337 = property class="Pnl"(reference=w865) -> ("Controls[]"=w863:refnum<vi>[])  [unwired: 1 in, 2 out]
            n338 = for {
              tunnel: w863 -> [w873] mode=indexing
              tunnel: [w870] -> w861 mode=indexing
              shift-right: [w869] -> w856
              shift-left: w857 -> [w869]
              n339 = property class="Ctl"(reference=w873) -> ("Label.Text"=w872:string, "Value"=w871:variant)  [unwired: 1 in, 2 out]
              n340 = Bundle("Label.Text"=w872, "Value"=w871) -> (w870:cluster{"Label.Text":string, "Value":variant})  [unwired: 1 in]
            }
            n341 = Bundle(cluster=w862, "All Control Values Variant"=w861) -> (w859:T3)  [unwired: 6 in]
            n342 = Bundle(cluster=w860, w859) -> (w858:cluster{"Time (s)":dbl, T3, bool})  [unwired: 2 in]
            n343 = Replace Array Subset(array=w868, new element=w858, index=w866) -> (w867:cluster{"Time (s)":dbl, T3, bool}[])
            n344 = Close Reference(reference=w856) -> ()  [unwired: 1 in, 1 out]
          }
        }
      }
      event "Inhale": Value Change {
        n345 = event-data() -> ()  [unwired: 1 in, 1 out]
        n346 = Unbundle(w884) -> ("Updated Waypoints"=w883:cluster{"x":dbl, "y":dbl, "th":dbl}[])  [unwired: 3 out]
        n347 = Unbundle(w882) -> ("Filename"=w881:string)  [unwired: 2 out]
        n348 = call "Find Command with Tag.vi"("Command Tag"=w881, "Commands"=w876) -> ("Index"=w878:i32, "Found Command"=w879:cluster{"Time (s)":dbl, T3, bool}, "Found"=w880:bool)  [unwired: 7 in]
        n349 = case shown="True" w880 {
          tunnel: w879 -> [_ w899]
          tunnel: w878 -> [_ w905]
          tunnel: w876 -> [w888 w907]
          tunnel: [w888 w906] -> w877
          tunnel: [_ TRUE] -> w875
          frame False {
          }
          frame True {
            n350 = Unbundle(w899) -> (w901:T3)  [unwired: 2 out]
            n351 = Unbundle(w901) -> ("Path"=w890:path)  [unwired: 6 out]
            n352 = call "Localize Path.vi"("Path"=w890) -> ("Local path"=w889:path)
            n353 = Open VI Reference(vi path=w889) -> (vi reference=w903:refnum<vi>)  [unwired: 5 in, 1 out]
            n354 = property class="VI"(reference=w903) -> (reference out=w896:refnum<vi>, "Panel"=w904:refnum<vi>)  [unwired: 1 in, 1 out]
            n355 = property class="Pnl"(reference=w904) -> (reference out=w894:refnum<vi>, "Controls[]"=w902:refnum<vi>[])  [unwired: 1 in, 1 out]
            n356 = for {
              tunnel: w902 -> [w913] mode=indexing
              tunnel: [w910] -> w900 mode=indexing
              shift-right: [w909] -> w892
              shift-left: w896 -> [w909]
              shift-right: [w908] -> _
              shift-left: w894 -> [w908]
              n357 = property class="Ctl"(reference=w913) -> ("Label.Text"=w912:string, "Value"=w911:variant)  [unwired: 1 in, 2 out]
              n358 = Bundle("Label.Text"=w912, "Value"=w911) -> (w910:cluster{"Label.Text":string, "Value":variant})  [unwired: 1 in]
            }
            n359 = Bundle(cluster=w901, "All Control Values Variant"=w900) -> (w898:T3)  [unwired: 6 in]
            n360 = Bundle(cluster=w899, w898) -> (w897:cluster{"Time (s)":dbl, T3, bool})  [unwired: 2 in]
            n361 = Replace Array Subset(array=w907, new element=w897, index=w905) -> (w906:cluster{"Time (s)":dbl, T3, bool}[])
            n362 = property class="VI"(reference=w892, "FP.State"=T23."Closed" ("Front Panel Window:State")) -> (reference out=w891:refnum<vi>)  [unwired: 1 in, 1 out]
            n363 = Close Reference(reference=w891) -> ()  [unwired: 1 in, 1 out]
          }
        }
      }
      event "fps": Cursor Move {
        n364 = event-data() -> ("CursIdx"=w916:i32, "CursLoc"=w922:cluster{"X":dbl, "Y":dbl})  [unwired: 1 in]
        n365 = Unbundle(w923) -> ("Updated Waypoints"=w921:cluster{"x":dbl, "y":dbl, "th":dbl}[])  [unwired: 3 out]
        n366 = Array Size(array=w919) -> (size(s)=w918:i32)
        n367 = Greater?(x=w918, y=w916) -> (0:w917:bool)
        n368 = case shown="False" w917 {
          tunnel: w922 -> [w930 w935]
          tunnel: w919 -> [w928 w933]
          tunnel: [w928 w932] -> w920
          tunnel: w916 -> [_ w931]
          frame False {
            n369 = Unbundle(w930) -> ("X"=w929:dbl)  [unwired: 1 out]
            n370 = local write "Time (s)"(w929) -> ()
          }
          frame True {
            n371 = Unbundle(w935) -> ("X"=w934:dbl)  [unwired: 1 out]
            n372 = in-place {
              in-place-border: w934 -> [w938]
              n373 = in-place-array #2(w933, w931) -> (w937:cluster{"Time (s)":dbl, T3, bool})
              n374 = Bundle(cluster=w937, "Time (s)"=w938) -> (w936:cluster{"Time (s)":dbl, T3, bool})  [unwired: 2 in]
              n375 = in-place-array #2(w936) -> (w932:cluster{"Time (s)":dbl, T3, bool}[])  [unwired: 1 out]
            }
          }
        }
      }
      event "Command Sequence": Mouse Down {
        # "click on enable of row ?"
        n376 = event-data() -> ("CtlRef"=w953:refnum<vi>, "Coords"=w954:T30, "PlatMods.Shift"=w939:bool)  [unwired: 1 in]
        n377 = Unbundle(w956) -> ("Updated Waypoints"=w955:cluster{"x":dbl, "y":dbl, "th":dbl}[])  [unwired: 3 out]
        n378 = invoke class="Tree (strict)" method="Point To Row Column"(reference=w953, "Point"=w954) -> ("Tag"=w944:string, "Col"=w948:i32)  [unwired: 6 in, 6 out]
        n379 = String Subset(string=w944, length (rest)=2 ("length (rest)")) -> (substring=w952:string)  [unwired: 1 in]
        n380 = Equal?(x=2 ("length (rest)"), y=w948) -> (x = y?=w947:bool)
        n381 = Equal?(x="//", y=w952) -> (x = y?=w946:bool)
        n382 = And(x=w946, y=w947) -> (x .and. y?=w945:bool)
        n383 = case shown="False" w945 {
          tunnel: w943 -> [w961 w964]
          tunnel: w944 -> [_ w968]
          tunnel: [w961 w963] -> w941
          tunnel: [_ TRUE] -> w942
          tunnel: w939 -> [_ w962]
          frame False {
          }
          frame True {
            n384 = call "Find Command with Tag.vi"("Command Tag"=w968, "Commands"=w964) -> ("Index"=w965:i32, "Found Command"=w966:cluster{"Time (s)":dbl, T3, bool}, "Found"=w967:bool)  [unwired: 7 in]
            n385 = case shown="False" w962 {
              tunnel: w967 -> [w974 _]
              tunnel: w966 -> [w973 _]
              tunnel: w965 -> [w972 w983]
              tunnel: w964 -> [w971 w986]
              tunnel: [w970 w985] -> w963
              frame False {
                # "Toggle"
                n386 = case shown="True" w974 {
                  tunnel: w973 -> [_ w977]
                  tunnel: w972 -> [_ w980]
                  tunnel: w971 -> [w975 w981]
                  tunnel: [w975 w978] -> w970
                  frame False {
                  }
                  frame True {
                    n387 = Unbundle(w977) -> (w976:bool)  [unwired: 2 out]
                    n388 = Not(x=w976) -> (.not. x?=w982:bool)
                    n389 = Bundle(cluster=w977, w982) -> (w979:cluster{"Time (s)":dbl, T3, bool})  [unwired: 2 in]
                    n390 = Replace Array Subset(array=w981, new element=w979, index=w980) -> (w978:cluster{"Time (s)":dbl, T3, bool}[])
                  }
                }
              }
              frame True {
                # "Delete"
                n391 = Delete From Array(array=w986, length=1, index=w983) -> (array with subset deleted=w985:cluster{"Time (s)":dbl, T3, bool}[])  [unwired: 1 out]
              }
            }
          }
        }
      }
      event "Command Sequence": Double Click {
        n392 = event-data() -> ("CtlRef"=w1001:refnum<vi>, "Coords"=w1002:T30)  [unwired: 1 in]
        n393 = Unbundle(w1004) -> ("Updated Waypoints"=w1003:cluster{"x":dbl, "y":dbl, "th":dbl}[])  [unwired: 3 out]
        n394 = invoke class="Tree (strict)" method="Point To Row Column"(reference=w1001, "Point"=w1002) -> ("Tag"=w991:string, "Col"=w996:i32)  [unwired: 6 in, 6 out]
        n395 = String Subset(string=w991, length (rest)=2 ("length (rest)")) -> (substring=w1000:string)  [unwired: 1 in]
        n396 = Equal?(x=0 ("length (rest)"), y=w996) -> (x = y?=w995:bool)
        n397 = Equal?(x="//", y=w1000) -> (x = y?=w994:bool)
        n398 = And(x=w994, y=w995) -> (x .and. y?=w993:bool)
        n399 = case shown="True" w993 {
          tunnel: w992 -> [_ w1012]
          tunnel: w991 -> [_ w1010]
          tunnel: [_ w1009] -> w988
          frame False {
          }
          frame True {
            n400 = call "Open Command Panel.vi"("Commands"=w1012, "Tag"=w1010) -> ("Found"=w1011:bool)  [unwired: 9 in]
            n401 = Select(t=w1010, s=w1011, f="") -> (s? t:f=w1009:string)
          }
        }
        n402 = Bundle(cluster=w989, "Filename"=w988) -> (w990:T15)  [unwired: 2 in]
      }
      event "Command Sequence": Edit Cell? {
        n403 = event-data() -> ("String"=w1020:string, "Tag"=w1019:string, "Col"=w1022:i32)  [unwired: 1 in, 2 out]
        n404 = Unbundle(w1029) -> ("Updated Waypoints"=w1028:cluster{"x":dbl, "y":dbl, "th":dbl}[])  [unwired: 3 out]
        n405 = Equal?(x=1 ("length (rest)"), y=w1022) -> (x = y?=w1023:bool)
        n406 = String Subset(string=w1019, length (rest)=2 ("length (rest)")) -> (substring=w1027:string)  [unwired: 1 in]
        n407 = Equal?(x="//", y=w1027) -> (x = y?=w1024:bool)
        n408 = And(x=w1024, y=w1023) -> (x .and. y?=w1021:bool)
        n409 = case shown="False" w1021 {
          tunnel: [TRUE _] -> w1014
          tunnel: w1020 -> [_ w1043]
          tunnel: w1016 -> [w1034 w1040]
          tunnel: w1019 -> [_ w1039]
          tunnel: [w1034 w1041] -> w1017
          frame False {
          }
          frame True {
            n410 = call "Find Command with Tag.vi"("Command Tag"=w1039, "Commands"=w1040) -> ("Index"=w1037:i32, "Found Command"=w1036:cluster{"Time (s)":dbl, T3, bool}, "Found"=w1038:bool)  [unwired: 7 in]
            n411 = Scan From String(input string=w1043) -> (output 1=w1042:dbl)  [unwired: 4 in, 3 out]
            n412 = case shown="False" w1038 {
              tunnel: w1040 -> [w1044 w1047]
              tunnel: [w1044 w1048] -> w1041
              tunnel: w1042 -> [_ w1049]
              tunnel: w1037 -> [_ w1045]
              tunnel: w1036 -> [_ w1050]
              frame False {
              }
              frame True {
                n413 = Bundle(cluster=w1050, "Time (s)"=w1049) -> (w1046:cluster{"Time (s)":dbl, T3, bool})  [unwired: 2 in]
                n414 = Replace Array Subset(array=w1047, new element=w1046, index=w1045) -> (w1048:cluster{"Time (s)":dbl, T3, bool}[])
              }
            }
          }
        }
        n415 = event-data("Discard?"=w1014) -> ()  [unwired: 1 in, 1 out]
        n416 = Not(x=w1014) -> (.not. x?=w1015:bool)
      }
      event "Command Palette": Mouse Move {
        n417 = event-data() -> ("Coords"=w1058:T30)  [unwired: 1 in]
        n418 = Unbundle(w1061) -> ("Updated Waypoints"=w1060:cluster{"x":dbl, "y":dbl, "th":dbl}[])  [unwired: 3 out]
        n419 = control-ref of="Command Palette"() -> (w1054:refnum<vi>)
        n420 = Unbundle(w1051) -> ("Filtered Command Info Out"=w1056:T2, "2D Picture"=w1059:picture)
        n421 = call "Picture Coord to Row.vi"("Row Height"=w1053, "Coords"=w1058, "Picture in"=w1054) -> ("Row Index"=w1055:i32, "Clicked in canvas"=w1057:bool)  [unwired: 7 in]
        n422 = case shown="True" w1057 {
          tunnel: w1059 -> [_ w1069]
          tunnel: w1056 -> [_ _]
          tunnel: w1053 -> [_ w1067]
          tunnel: w1055 -> [_ w1066]
          frame False {
          }
          frame True {
            n423 = Multiply(x=w1066, y=w1067) -> (x*y=w1072:i32)
            n424 = Add(x=w1072, y=w1067) -> (x+y=w1073:i32)
            n425 = Bundle(0, w1072, 300, w1073) -> (w1074:cluster{i32, i32, i32, i32})  [unwired: 1 in]
            n426 = call <vilib>:"Draw Rectangle.vi"("rect"=w1074, "fill?(F)"=TRUE, "color(black)"=u32 10539263) -> ("new picture"=w1076:picture)  [unwired: 6 in]
            n427 = Concatenate Strings(w1076, w1069) -> (→"Command Palette":picture)
          }
        }
      }
      event "Command Palette": Mouse Down {
        n428 = event-data() -> ("Coords"=w1088:T30, "Mods"=w1090:cluster{"Double Click":bool, "Menu Key":bool})  [unwired: 1 in, 1 out]
        n429 = control-ref of="Command Palette"() -> (w1089:refnum<vi>)
        n430 = Unbundle(w1092) -> ("Updated Waypoints"=w1091:cluster{"x":dbl, "y":dbl, "th":dbl}[])  [unwired: 3 out]
        n431 = call "Picture Coord to Row.vi"("Row Height"=w1087, "Coords"=w1088, "Picture in"=w1089) -> ("Row Index"=w1083:i32, "Clicked in canvas"=w1086:bool)  [unwired: 7 in]
        n432 = Unbundle(w1090) -> ("Double Click"=w1085:bool)  [unwired: 1 out]
        n433 = Unbundle(w1078) -> ("Filtered Command Info Out"=w1082:T2)  [unwired: 1 out]
        n434 = Compound Arithmetic op=AND(w1086, w1085) -> (w1084:bool)
        n435 = case shown="True" w1084 {
          tunnel: w1083 -> [_ w1105]
          tunnel: w1082 -> [_ w1106]
          tunnel: w1080 -> [w1097 w1101]
          tunnel: [w1097 w1098] -> w1081
          frame False {
          }
          frame True {
            n436 = local read "Time (s)"() -> (w1102:dbl)
            n437 = Index Array(array=w1106, index=w1105) -> (element=w1104:T3)
            n438 = for {
              tunnel: w1101 -> [w1111] mode=indexing
              tunnel: w1102 -> [w1109]
              tunnel: [w1107] -> w1099
              i -> [w1107]
              stop <- w1108 stop-if-true
              n439 = Unbundle(w1111) -> ("Time (s)"=w1110:dbl)  [unwired: 2 out]
              n440 = Greater Or Equal?(x=w1110, y=w1109) -> (x >= y?=w1108:bool)
            }
            n441 = Bundle("Time (s)"=w1102, w1104, TRUE) -> (w1100:cluster{"Time (s)":dbl, T3, bool})  [unwired: 1 in]
            n442 = Insert Into Array(array=w1101, index=w1099, new element=w1100) -> (w1098:cluster{"Time (s)":dbl, T3, bool}[])
          }
        }
      }
    }
    n443 = feedback-in #1(w77) -> ()
    n444 = flat-sequence {
      tunnel: ["Time (s)"] -> w99
      tunnel: ["Sample Period (s)"] -> w56
      tunnel: ["Limits"] -> w83
      tunnel: ["Conditions"] -> w80
      tunnel: [w108] -> w45
      tunnel: ["Acceleration Overrides"] -> w72
      tunnel: w71 -> [_]
      tunnel: w49 -> [w108]
      tunnel: w48 -> [w107]
      frame #0 {
        n445 = control-ref of="Command Sequence"() -> (w109:refnum<vi>)
        n446 = call "Format Tree.vi"("Update"=w107, "Commands"=w108, "Tree Refnum"=w109) -> ()  [unwired: 9 in]
      }
    }
    n447 = control-ref of="Acceleration Overrides"() -> (w70:refnum<vi>)
    n448 = call "Enforce Robot Rules.vi"("Clust Refnum"=w70, "Disable"=w91, "New Points"=w93, "Original Points"=w92) -> ("Points out"=w71:cluster{"x":dbl, "y":dbl, "th":dbl}[])  [unwired: 7 in]
    "WayPoints" <- w71
    n449 = Divide(x=w99, y=w56) -> (x/y=w90:dbl)
    n450 = Bundle("Sample Period (s)"=w56, "Limits"=w83, "Conditions"=w80, "Acceleration Overrides"=w72) -> (w79:T24)  [unwired: 1 in]
    n451 = call "GenNewTraj.vi"("Parameters"=w79, "Points in"=w71) -> ("Time (s)"=w78:dbl, "Valid"=w57:bool, "Trajectory Data"=w69:T12, "Updated Waypoints"=w81:cluster{"x":dbl, "y":dbl, "th":dbl}[], "Distance (ft)"=w82:dbl)  [unwired: 5 in]
    "Duration (s)" <- w78
    "Distance (ft)" <- w82
    n452 = property on="Time (s)" class="Slide (strict)"("Scale.Maximum"=w78) -> ()  [unwired: 2 in, 2 out]
    n453 = Bundle("Time (s)"=w78, "Distance (ft)"=w82) -> (w95:cluster{"Time (s)":dbl, "Distance (ft)":dbl})  [unwired: 1 in]
    n454 = Bundle("Trajectory Data"=w69, "Updated Waypoints"=w81, w79, w45) -> (w74:T37)  [unwired: 1 in]
    n455 = call "Draw Trajectory.vi"("Robot Index"=w90, "new picture in"=picture data[5B] ("new picture"), "Trajectory Data"=w69, "Picture in"=w102) -> ("Path Points"=w84:cluster{"x":dbl, "y":dbl}[], "Output Point"=w98:T38, "new picture"=w100:picture)  [unwired: 5 in]
    n456 = Unbundle(w67) -> ("Hover Object"=w66:T14)  [unwired: 2 out]
    n457 = call "Draw Shapes.vi"("Path Points"=w84, "Sample Period (s)"=w56, "Output Point"=w98, "Commands"=w45, "Results"=w66, "new picture in"=w100, "Points"=w81, "Picture in"=w102) -> ("new picture out"=→"Picture":picture)  [unwired: 3 in]
    n458 = call "Saved Checker.vi"("comp A"=w85, "comp B"=w74) -> ("Unsaved"=w41:bool)
    n459 = call "Update Annotations.vi"("Sample Period"=w56, "Commands"=w45, "Trajectory Data"=w69, "Robot Pt Index"=w90) -> ("Redraw"=w47:bool, "Velocity Trace"=w46:dbl[], "Annotation Data"=w89:T39)  [unwired: 5 in]
    n460 = Select(t=0, s=w61, f=2000) -> (s? t:f=w62:i32)
    n461 = Select(t=cluster{u32, u32}[] [{14869218, 14869218}] ("Colors [4]"), s=w57, f=cluster{u32, u32}[] [{6094681, 6094681}] ("Colors [4]")) -> (s? t:f=w60:cluster{u32, u32}[])
    n462 = case shown="True" w47 {
      tunnel: w89 -> [_ w106]
      tunnel: w46 -> [_ w105]
      frame False {
      }
      frame True {
        n463 = property on="fps" class="WFGraph (strict)"("AnntList"=w106) -> ()  [unwired: 2 in, 2 out]
        "fps" <- w105
      }
    }
    n464 = Select(t=u32 16711680 ("Boolean Text.Text Colors:Text Color"), s=w41, f=u32 0 ("Boolean Text.Text Colors:Text Color")) -> (s? t:f=w42:u32)
    n465 = property on="Unjank" class="Bool"("Colors [4]"=w60) -> ()  [unwired: 2 in, 2 out]
    n466 = property on="Save" class="Bool"("BoolText.TextColor"=w42) -> ()  [unwired: 2 in, 2 out]
  }
  n467 = Format Into String(format string=w19, w1) -> (resulting string=w20:string)  [unwired: 2 in, 1 out]
  n468 = property class="VI"("Front Panel.Title"=w20) -> ()  [unwired: 2 in, 2 out]
  n469 = event shown="[0] Timeout" {
    selector: _ -> [_]
    dyn-events: _ -> [_]
    timeout: _ -> [_]
    event Timeout {
      n470 = event-data() -> ()  [unwired: 1 in, 3 out]
    }
  }
